vi "MarvinATP1.vi"() -> ()   [LabVIEW 2017]
uses:
  PCAN_Driver/ControlCAN.llb/InitFlag.ctl
  PCAN_Driver/ControlCAN.lvlib
  PCAN_Driver/ControlCAN.llb/Mode.ctl
  PCAN_Driver/ControlCAN.llb/Fliter.ctl
  PCAN_Driver/ControlCAN.llb/VCI_INIT_CONFIG.ctl
  PCAN_Driver/ControlCAN.llb/CAN Channel.ctl
  PCAN_Driver/ControlCAN.llb/DevType.ctl
panel:
  out "Auxiind":bool
  in  "Index":string="5"
  out "Array 2":dbl[](array[numeric])
  out "Array 3":string[](array[string])
  out "Array 4":dbl[](array[numeric])
  out "Array 5":dbl[](array[numeric])
  out "TempSensCalind":bool
  out "VisualInspectionResult":bool
  in  "Stop Burn-in":bool
  out "Burninind":bool
  out "TempControlind":bool
  out "TempAlg":bool=TRUE
  out "MotorTempind":bool
  out "SpeedStopind":bool
  out "VC15100-1 Vel":dbl
  out "VC15100-1 Cur":dbl
  out "VC1500-2 Vel":dbl
  out "VC15100-2":dbl
  out "EnableTestind":bool
  out "ComTestind":bool
  out "Ambient Temperature":dbl
  out "Motor Speed RPM":dbl
  out "Motor Stator Temp.":dbl
  out "Power transistor Heat sink Temp.":dbl
  in  "ATR":string[][](table)=[["Test Communication", "-", "-", "-", "-", ""], ["Set S/N", "-", "-", "-", "-", ""], ["Set Board Number", "-", "-", "-", "-", ""], [" ", "", "", "", "", ""], ["Test Communication", "-", "-", "-", "-", ""], ["Get S/N", "-", "-", "-", "", ""], ["Get Board Number", "-", "-", "-", "", ""], ["Get FW", "-", "-", "-", "", ""], ["Enable Motor", "", "", "", "", ""], ["Small position command", "", "", "", "", ""], ["Measure delta", "", "", "", "", ""], ["Velocity command", "", "", "", "", ""]]
  out "Pannel User Message":string
  out "Config_CANAT":T7 {"DevType" items=["USB-CAN"=3, "USB-CAN2"=4]; "CanIndex" items=["通道1", "通道2"]; "VCI_INIT_CONFIG"."Fliter" items=["接收所有类型"=3, "只接收标准帧"=4, "只接收扩展帧"=7]; "VCI_INIT_CONFIG"."Mode" items=["正常工作", "自测模式（环回）", "仅侦听模式"]; "VCI_INIT_CONFIG"."InitFlag" items=["使用Flash参数", "使用界面设置参数"]}
  in  "Stop Button":bool
  out "UUT":u8
  out "VISA resource name out":refnum<visa-resource-name>
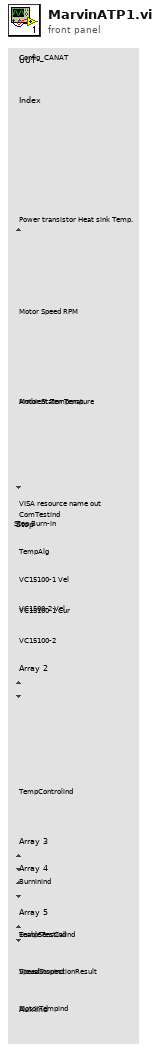
[diagram p1: front panel]
types:
  T1 = typedef "ControlCAN.lvlib/DevType.ctl" = u32
  T2 = typedef "ControlCAN.lvlib/CAN Channel.ctl" = u32
  T3 = typedef "ControlCAN.lvlib/VCI_INIT_CONFIG.ctl" = cluster{"AccCode":u32, "AccMask":u32, "InitFlag":T4, "Fliter":T5, "Timing0":u8, "Timing1":u8, "Mode":T6}
  T4 = typedef "ControlCAN.lvlib/InitFlag.ctl" = u32
  T5 = typedef "ControlCAN.lvlib/Fliter.ctl" = u8
  T6 = typedef "ControlCAN.lvlib/Mode.ctl" = u8
  T7 = cluster{"DevType":T1, "DevIndex":u32, "CanIndex":T2, "VCI_INIT_CONFIG":T3}
  T8 = enum16{"STOP", "VC15100-2", "RESET", "VC15100-1", "MD0"}
  T9 = enum8{"Enabled", "Disabled", "Disabled and Grayed Out"}
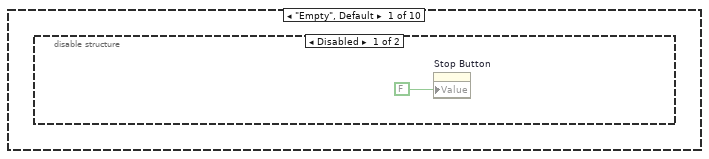
[diagram p2: hidden frame]
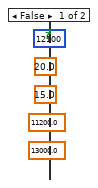
[diagram p6: hidden frame]
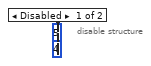
[diagram p7: hidden frame]
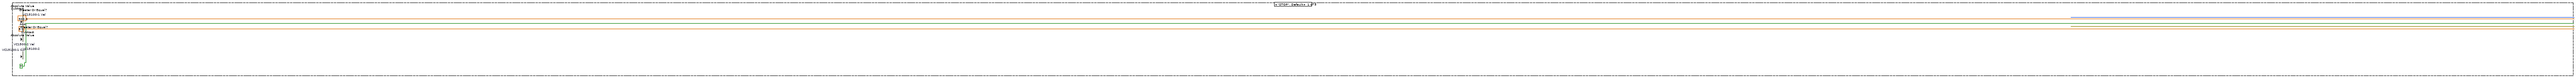
[diagram p8: hidden frame]
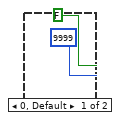
[diagram p9: hidden frame]
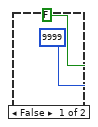
[diagram p10: hidden frame]
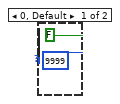
[diagram p11: hidden frame]
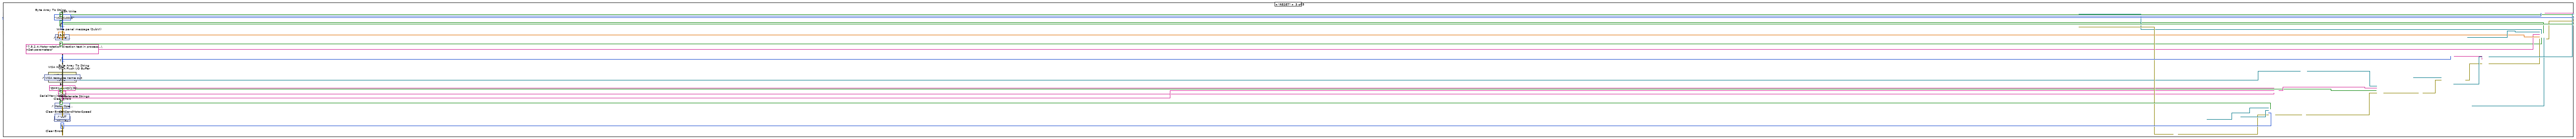
[diagram p13: hidden frame]
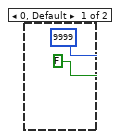
[diagram p15: hidden frame]
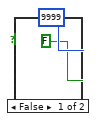
[diagram p16: hidden frame]
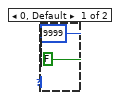
[diagram p17: hidden frame]
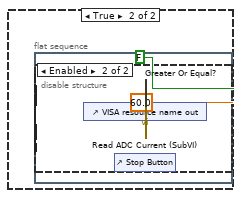
[diagram p18: hidden frame]
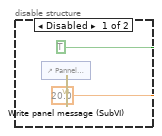
[diagram p19: hidden frame]
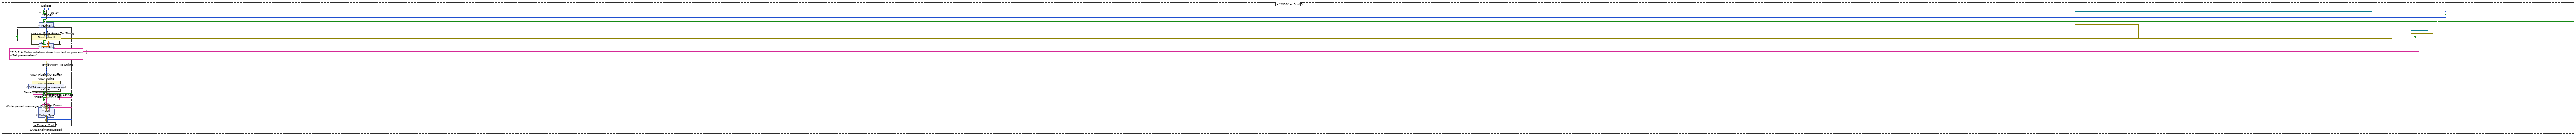
[diagram p20: hidden frame]
diagram:
  n1 = case shown="\"Auxiliary\"" {
    selector: _ -> [_ _ _ _ _ _ _ _ _ _]
    tunnel: _ -> [_ _ _ _ _ _ _ _ w1694 _]
    tunnel: _ -> [_ w34 w53 w705 w901 w1020 w1342 w1653 w1656 w1901]
    tunnel: _ -> [_ w14 w69 w710 w908 w1032 w1368 w1649 w1689 w1910]
    frame "Empty", Default {
      n2 = disable-structure shown="Disabled" {
        frame Disabled {
          n3 = property on="Stop Button" class="Bool (strict)"("Value"=FALSE ("Stop Button")) -> ()  [unwired: 2 in, 2 out]
        }
        frame Enabled {
        }
      }
    }
    frame "Com Test" {
      w11 = T9."Enabled" ("Disabled")
      w12 = T9."Disabled and Grayed Out" ("Disabled")
      w35 = 6 ("disabled index (col)")
      w4 = "7.4" ("Test Paragraph")
      n4 = control-ref of="Pannel User Message"() -> (w32:refnum<vi>)
      n5 = property on="Property Node" class="Bool (strict)"(error in=w14, "DisabledEnum"=w12) -> (error out=w13:errorcluster)  [unwired: 1 in, 1 out]
      n6 = property class="Str"(reference=w32, error in=w14, "Value"="7.4.Communication Test in process...") -> (error out=w3:errorcluster)  [unwired: 1 out]
      n7 = property on="Property Node" class="Bool (strict)"(error in=w13, "DisabledEnum"=w12) -> ()  [unwired: 1 in, 2 out]
      n8 = control-ref of="ATR"() -> (w5:refnum<vi>)
      n9 = call "Reset old test Values (SubVI).vi"("error in"=w3, "Atr in"=w5, "Test Paragraph"=w4) -> ("error out"=w2:errorcluster)  [unwired: 8 in]
      n10 = call "Table_ScrollaBarMarvin.vi"("error in"=w2, "Line to focus"=w4, "reference in"=w34) -> ("error out"=w33:errorcluster)  [unwired: 2 out]
      n11 = property on="Property Node" class="VISAName"() -> ("Value"=w29:refnum<visa-resource-name>)  [unwired: 2 in, 2 out]
      n12 = property on="Property Node" class="Str"() -> ("Value"=w18:string)  [unwired: 2 in, 2 out]
      n13 = control-ref of="UUT"() -> (w45:refnum<vi>)
      n14 = property class="Tbl (strict)"(reference=w34, error in=w33) -> (reference out=w22:refnum<vi>, error out=w49:errorcluster, "Value"=w6:string[][])
      n15 = Index Array(array=w6, index (col)=0 ("disabled index (col)")) -> (element=w50:string[])  [unwired: 1 in]
      n16 = call "Find_Number_LineMARVIN.vi"("Test Paragraph"=w4, "error in"=w49, "Row Headers[]"=w50) -> ("error out"=w47:errorcluster, "Line number"=w46:i32)  [unwired: 2 in, 2 out]
      n17 = call <vilib>:"Clear Errors.vi"("error in (no error)"=w47) -> ("error out"=w8:errorcluster)  [unwired: 5 in, 1 out]
      n18 = call "Time Delay"("error in (no error)"=w8) -> ("error out"=w7:errorcluster)  [unwired: 10 in]
      n19 = VISA Flush I/O Buffer(VISA resource name=w29, error in (no error)=w7) -> (VISA resource name out=w27:refnum<visa-resource-name>, error out=w28:errorcluster)  [unwired: 1 in]
      n20 = call "SerialMarvinMod.vi"("error in (no error)"=w28, "write buffer"="VR\r\n", "VISA resource name"=w27) -> ("error out"=w21:errorcluster, "read buffer"=w24:string)  [unwired: 7 in]
      n21 = Equal?(x=w18, y=w24) -> (x = y?=w16:bool)
      n22 = Increment(x=w46) -> (x+1=w26:i32)
      n23 = Increment(x=w26) -> (x+1=w37:i32)
      n24 = Replace Array Subset(array=w6, new element=w24, index (row)=w26, index (col)=5 ("disabled index (col)")) -> (w23:string[][])
      n25 = property class="Tbl (strict)"(reference=w22, error in=w21, "Value"=w23) -> (error out=w20:errorcluster)  [unwired: 1 out]
      n26 = call "PassOrFail (SubVI).vi"("disabled index (col)"=w35, "index (row)"=w26, "error in (no error)"=w20, "Boolean"=w16, "Table in"=w34) -> ("error out"=w19:errorcluster)  [unwired: 6 in]
      n27 = property class="DigNum (strict)"(reference=w45, error in=w19) -> (error out=w36:errorcluster, "Value"=w44:u8)  [unwired: 1 out]
      n28 = Equal?(x=w44, y=u8 47) -> (x = y?=w40:bool)
      n29 = Equal?(x=w44, y=u8 63) -> (x = y?=w39:bool)
      n30 = Equal?(x=w44, y=u8 95) -> (x = y?=w38:bool)
      n31 = Compound Arithmetic op=OR(w40, w39, w38) -> (w17:bool)
      n32 = call "PassOrFail (SubVI).vi"("disabled index (col)"=w35, "index (row)"=w37, "error in (no error)"=w36, "Boolean"=w17, "Table in"=w34) -> ("error out"=w9:errorcluster)  [unwired: 6 in]
      n33 = property on="Property Node" class="Bool (strict)"(error in=w9, "DisabledEnum"=w11) -> (error out=w10:errorcluster)  [unwired: 1 in, 1 out]
      n34 = property on="Property Node" class="Bool (strict)"(error in=w10, "DisabledEnum"=w11) -> ()  [unwired: 1 in, 2 out]
      n35 = And(x=w17, y=w16) -> (x .and. y?=→"ComTestind":bool)
    }
    frame "Enable Test" {
      w68 = T9."Enabled" ("Disabled")
      w71 = T9."Disabled and Grayed Out" ("Disabled")
      w52 = "7.5.2" ("Test Paragraph")
      n36 = control-ref of="Pannel User Message"() -> (w87:refnum<vi>)
      n37 = property on="Property Node" class="Bool (strict)"(error in=w69, "DisabledEnum"=w71) -> (error out=w70:errorcluster)  [unwired: 1 in, 1 out]
      n38 = property class="Str"(reference=w87, error in=w69, "Value"="7.5.2.Enable Test") -> (error out=w86:errorcluster)  [unwired: 1 out]
      n39 = property on="Property Node" class="Bool (strict)"(error in=w70, "DisabledEnum"=w71) -> ()  [unwired: 1 in, 2 out]
      n40 = call "Table_ScrollaBarMarvin.vi"("error in"=w86, "Line to focus"=w52, "reference in"=w53) -> ("error out"=w125:errorcluster)  [unwired: 2 out]
      n41 = call "Reset old test Values (SubVI).vi"("error in"=w125, "Atr in"=w53, "Test Paragraph"=w52) -> ("error out"=w54:errorcluster)  [unwired: 8 in]
      n42 = property class="Tbl (strict)"(reference=w53, error in=w54) -> (error out=w127:errorcluster, "Value"=w128:string[][])  [unwired: 1 out]
      n43 = control-ref of="VISA resource name out"() -> (w98:refnum<vi>)
      n44 = property on="Property Node" class="Str"() -> ("Value"=w62:string)  [unwired: 2 in, 2 out]
      n45 = control-ref of="Stop Button"() -> (w64:refnum<vi>)
      n46 = control-ref of="Config_CANAT"() -> (w80:refnum<vi>)
      n47 = control-ref of="UUT"() -> (w81:refnum<vi>)
      n48 = Initialize Array(FALSE, 14 ("dimension size")) -> (w110:bool[])
      n49 = Build Array (concatenate)(w110, bool[] [FALSE, FALSE, FALSE, FALSE, FALSE, FALSE, FALSE] ("array")) -> (w111:bool[])
      n50 = Boolean Array To Number(Boolean array=w111) -> (number=w109:u32)
      n51 = To Unsigned Long Integer(number=w109) -> (unsigned 32bit integer=w100:u32)
      n52 = Split Number(x=w100) -> (hi(x)=w105:u16, lo(x)=w106:u16)
      n53 = Split Number(x=w106) -> (hi(x)=w104:u8, lo(x)=w103:u8)
      n54 = Index Array(array=w128, index (col)=0 ("disabled index (col)")) -> (element=w129:string[])  [unwired: 1 in]
      n55 = Equal?(x=w62, y="EBAY") -> (x = y?=w60:bool)
      n56 = case shown="True" w60 {
        tunnel: [u16 12100 ("Motor Speed RPM") u16 15100 ("Motor Speed RPM")] -> w59
        tunnel: [11200.0 ("y") 14800.0 ("y")] -> w58
        tunnel: [13000.0 ("y") 16000.0 ("y")] -> w57
        tunnel: [20.0 ("y") 48.0 ("y")] -> w56
        tunnel: [15.0 ("y") 40.0 ("y")] -> w55
        frame False {
        }
        frame True {
        }
      }
      n57 = call "Find_Number_LineMARVIN.vi"("Test Paragraph"=w52, "error in"=w127, "Row Headers[]"=w129) -> ("error out"=w63:errorcluster, "Line number"=w124:i32)  [unwired: 2 in, 2 out]
      n58 = for {
        tunnel: w53 -> [w663]
        tunnel: w124 -> [w653]
        tunnel: u16[] [5000, 0, 5000] -> [w628] mode=indexing
        tunnel: [w651] -> w122
        tunnel: w63 -> [w629]
        tunnel: bool[] [TRUE, FALSE, TRUE] -> [w627] mode=indexing
        tunnel: bool[] [TRUE, TRUE, TRUE] -> [w626] mode=indexing
        tunnel: [w625] -> w77 mode=indexing
        i -> [w655]
        w656 = 200.0 ("y")
        n59 = control-ref of="VISA resource name out"() -> (w648:refnum<vi>)
        n60 = control-ref of="Config_CANAT"() -> (w670:refnum<vi>)
        n61 = while {
          tunnel: [w675] -> w665
          tunnel: [w692] -> w664
          tunnel: w622 -> [w691]
          tunnel: w624 -> [w689]
          stop <- w674 stop-if-true
          w686 = 15.0 ("y")
          n62 = control-ref of="Motor Speed RPM"() -> (w693:refnum<vi>)
          n63 = control-ref of="Pannel User Message"() -> (w687:refnum<vi>)
          n64 = flat-sequence {
            tunnel: [w694] -> w690
            frame #0 {
              n65 = call <vilib>:"High Resolution Relative Seconds.vi"() -> ("relative seconds"=w694:dbl)
            }
          }
          n66 = property on="Stop Button" class="Bool (strict)"() -> ("Value"=w673:bool)  [unwired: 2 in, 2 out]
          n67 = Subtract(x=w690, y=w689) -> (x-y=w685:dbl)
          n68 = Greater Or Equal?(x=w685, y=w686) -> (x >= y?=w688:bool)
          n69 = Compound Arithmetic op=OR(w673, w688) -> (w674:bool)
          n70 = Subtract(x=w686, y=w685) -> (x-y=w677:dbl)
          n71 = Number To Fractional String(number=w677, precision (6)=i16 2) -> (F-format string=w683:string)  [unwired: 2 in]
          n72 = property class="DigNum (strict)"(reference=w693, error in=w691) -> (error out=w692:errorcluster, "Value"=w675:dbl)  [unwired: 1 out]
          n73 = Number To Decimal String(number=w675) -> (decimal integer string=w684:string)  [unwired: 1 in]
          n74 = Concatenate Strings("7.5.2.Enable Test in process...\nRemained Time: " ("string"), w683, "  sec." ("string"), "\r\n", "Motor speed [rpm]: " ("string"), w684) -> (w678:string)
          n75 = property class="Str"(reference=w687, "Value"=w678) -> ()  [unwired: 1 in, 2 out]
        }
        n76 = Add(x=w628, y=w656) -> (x+y=w658:dbl)
        n77 = Increment(x=w655) -> (x+1=w654:i32)
        n78 = flat-sequence {
          tunnel: [w672] -> w624
          tunnel: w623 -> [w671]
          tunnel: [w671] -> w622
          frame #0 {
            n79 = call <vilib>:"High Resolution Relative Seconds.vi"() -> ("relative seconds"=w672:dbl)
          }
        }
        n80 = Subtract(x=w628, y=w656) -> (x-y=w657:dbl)
        n81 = In Range and Coerce(upper limit=w658, x=w665, lower limit=w657) -> (In Range?=w625:bool)  [unwired: 1 out]
        n82 = Add(x=w653, y=w654) -> (x+y=w650:i32)
        n83 = case shown="True" w627 {
          tunnel: [bool[] [FALSE, FALSE, FALSE, FALSE, FALSE, FALSE, FALSE] ("array") bool[] [FALSE, FALSE, FALSE, TRUE, FALSE, FALSE, FALSE] ("array")] -> w635
          frame False {
          }
          frame True {
          }
        }
        n84 = call <vilib>:"Clear Errors.vi"("error in (no error)"=w664) -> ("error out"=w621:errorcluster)  [unwired: 5 in, 1 out]
        n85 = call "PassOrFail (SubVI).vi"("disabled index (col)"=6, "index (row)"=w650, "error in (no error)"=w621, "Boolean"=w625, "Table in"=w663) -> ("error out"=w667:errorcluster)  [unwired: 6 in]
        n86 = property class="Tbl (strict)"(reference=w663, error in=w667) -> (reference out=w659:refnum<vi>, error out=w668:errorcluster, "Value"=w660:string[][])
        n87 = Build Array (concatenate)(bool[] [FALSE, FALSE, FALSE, TRUE, FALSE, FALSE, FALSE, FALSE, FALSE, FALSE, FALSE, FALSE, FALSE, FALSE] ("array"), w635) -> (w636:bool[])
        n88 = Boolean Array To Number(Boolean array=w636) -> (number=w637:u32)
        n89 = To Unsigned Long Integer(number=w637) -> (unsigned 32bit integer=w646:u32)
        n90 = Split Number(x=w646) -> (hi(x)=w641:u16, lo(x)=w640:u16)
        n91 = Split Number(x=w640) -> (hi(x)=w642:u8, lo(x)=w643:u8)
        n92 = Number To Fractional String(number=w665, precision (6)=i16 2) -> (F-format string=w662:string)  [unwired: 2 in]
        n93 = Replace Array Subset(array=w660, new element=w662, index (row)=w650, index (col)=5 ("disabled index (col)")) -> (w661:string[][])
        n94 = property class="Tbl (strict)"(reference=w659, error in=w668, "Value"=w661) -> (error out=w651:errorcluster)  [unwired: 1 out]
        n95 = property class="VISAName"(reference=w648, error in=w629) -> (error out=w649:errorcluster, "Value"=w639:refnum<visa-resource-name>)  [unwired: 1 out]
        n96 = Split Number(x=w641) -> (hi(x)=w644:u8, lo(x)=w645:u8)
        n97 = Build Array(u8 75, u8 0 ("element"), u8 4 ("Length"), u8 2, w643, w642, w645, w644) -> (w638:u8[])
        n98 = Byte Array To String(unsigned byte array=w638) -> (string=w647:string)
        n99 = VISA Write(VISA resource name=w639, write buffer=w647, error in (no error)=w649) -> (error out=w630:errorcluster)  [unwired: 2 out]
        n100 = case shown="True" w626 {
          tunnel: w670 -> [_ w700]
          tunnel: [w695 w699] -> w623
          tunnel: w630 -> [w695 w697]
          frame False {
          }
          frame True {
            n101 = control-ref of="UUT"() -> (w701:refnum<vi>)
            n102 = call "CANSendMotorSpeed.vi"("Remote"=TRUE, "error in (no error)"=w697, "Motor Speed RPM"=u16 5000, "UUT"=w701, "Cluster in"=w700) -> ("error out"=w699:errorcluster)  [unwired: 6 in]
          }
        }
      }
      n103 = And Array Elements(Boolean array=w77) -> (logical AND=w76:bool)
      n104 = Split Number(x=w105) -> (hi(x)=w102:u8, lo(x)=w101:u8)
      n105 = Build Array(u8 75, u8 0 ("element"), u8 4 ("Length"), u8 2, w103, w104, w101, w102) -> (w108:u8[])
      n106 = Byte Array To String(unsigned byte array=w108) -> (string=w99:string)
      n107 = call <vilib>:"Clear Errors.vi"("error in (no error)"=w122) -> ("error out"=w73:errorcluster)  [unwired: 5 in, 1 out]
      n108 = disable-structure shown="Enabled" {
        disable-tunnel: w73 -> [w162 w618]
        disable-tunnel: [w161 w617] -> w79
        disable-tunnel: [w160 w619] -> w75
        disable-tunnel: T8."MD0" -> [w159 _]
        disable-tunnel: w64 -> [w158 _]
        disable-tunnel: w59 -> [w157 _]
        disable-tunnel: w58 -> [w156 _]
        disable-tunnel: w57 -> [w155 _]
        disable-tunnel: w56 -> [w154 _]
        disable-tunnel: w55 -> [w153 _]
        frame Enabled {
          n109 = while {
            tunnel: [w174] -> w160
            tunnel: w162 -> [w176]
            tunnel: [w175] -> w161
            shift-right: [w172] -> _
            shift-left: w159 -> [w173]
            tunnel: w158 -> [w168]
            tunnel: w157 -> [w167]
            tunnel: w156 -> [w166]
            tunnel: w155 -> [w165]
            tunnel: w154 -> [w164]
            tunnel: w153 -> [w163]
            stop <- w170 stop-if-true
            n110 = case shown="\"VC15100-2\"" w173 {
              selector: w173 -> [w190 _ _ _ _]
              tunnel: w176 -> [w191 w219 w373 w413 w579]
              tunnel: [w191 w212 w379 w407 w578] -> w175
              tunnel: [w183 FALSE FALSE FALSE FALSE] -> w174
              tunnel: [w190 T8."STOP" T8."VC15100-2" w399 w582] -> w172
              tunnel: [TRUE FALSE FALSE FALSE FALSE] -> w171
              tunnel: w168 -> [_ w198 w357 w393 w573]
              tunnel: w167 -> [_ w197 _ _ _]
              tunnel: w166 -> [_ w196 _ _ _]
              tunnel: w165 -> [_ w195 _ _ _]
              tunnel: w164 -> [_ w194 _ w391 _]
              tunnel: w163 -> [_ w193 _ w392 _]
              frame "STOP", Default {
                n111 = property on="VC15100-1 Vel" class="DigNum (strict)"() -> ("Value"=w182:dbl)  [unwired: 2 in, 2 out]
                n112 = property on="VC1500-2 Vel" class="DigNum (strict)"() -> ("Value"=w181:dbl)  [unwired: 2 in, 2 out]
                n113 = Subtract(x=w182, y=w181) -> (x-y=w180:dbl)
                n114 = Absolute Value(x=w180) -> (abs(x)=w179:dbl)
                n115 = Greater Or Equal?(x=w179, y=500.0) -> (x >= y?=w177:bool)
                n116 = property on="VC15100-2" class="DigNum (strict)"() -> ("Value"=w189:dbl)  [unwired: 2 in, 2 out]
                n117 = property on="VC15100-1 Cur" class="DigNum (strict)"() -> ("Value"=w188:dbl)  [unwired: 2 in, 2 out]
                n118 = Subtract(x=w189, y=w188) -> (x-y=w185:dbl)
                n119 = Absolute Value(x=w185) -> (abs(x)=w184:dbl)
                n120 = Greater Or Equal?(x=w184, y=5.0) -> (x >= y?=w186:bool)
                n121 = And(x=w177, y=w186) -> (x .and. y?=w183:bool)
              }
              frame "VC15100-2" {
                n122 = control-ref of="VISA resource name out"() -> (w214:refnum<vi>)
                n123 = property on="Property Node" class="DigNum (strict)"() -> ("Value"=w207:dbl)  [unwired: 2 in, 2 out]
                n124 = flat-sequence {
                  tunnel: [w313] -> w218
                  tunnel: w217 -> [w312]
                  tunnel: [w312] -> w216
                  frame #0 {
                    n125 = call <vilib>:"High Resolution Relative Seconds.vi"() -> ("relative seconds"=w313:dbl)
                  }
                }
                n126 = control-ref of="Config_CANAT"() -> (w221:refnum<vi>)
                n127 = control-ref of="UUT"() -> (w220:refnum<vi>)
                n128 = call <vilib>:"Clear Errors.vi"("error in (no error)"=w216) -> ("error out"=w206:errorcluster)  [unwired: 5 in, 1 out]
                n129 = while {
                  tunnel: w218 -> [w337]
                  tunnel: w206 -> [w331]
                  tunnel: [w332] -> w213
                  tunnel: [w330] -> w211
                  tunnel: w198 -> [w318]
                  tunnel: w196 -> [w315]
                  tunnel: w195 -> [w314]
                  stop <- w335 stop-if-true
                  w316 = "7.5.2.4.Motor rotation direction test in process..." ("string")
                  n130 = control-ref of="Motor Speed RPM"() -> (w317:refnum<vi>)
                  n131 = control-ref of="Pannel User Message"() -> (w326:refnum<vi>)
                  n132 = property class="DigNum (strict)"(reference=w317, error in=w331) -> (error out=w332:errorcluster, "Value"=w321:dbl)  [unwired: 1 out]
                  "VC1500-2 Vel" <- w321
                  n133 = Number To Fractional String(number=w321, precision (6)=i16 2) -> (F-format string=w325:string)  [unwired: 2 in]
                  n134 = Concatenate Strings(w316, "\r\n", "Motor speed [rpm]: " ("string"), w325) -> (w320:string)
                  n135 = property class="Str"(reference=w326, "Value"=w320) -> ()  [unwired: 1 in, 2 out]
                  n136 = Greater Or Equal?(x=w321, y=w315) -> (x >= y?=w329:bool)
                  n137 = call <vilib>:"High Resolution Relative Seconds.vi"() -> ("relative seconds"=w338:dbl)
                  n138 = Subtract(x=w338, y=w337) -> (x-y=w333:dbl)
                  n139 = Less Or Equal?(x=w321, y=w314) -> (x <= y?=w328:bool)
                  n140 = And(x=w329, y=w328) -> (x .and. y?=w327:bool)
                  n141 = case shown="True" w327 {
                    selector: w327 -> [w339 w344]
                    tunnel: [w339 w343] -> w330
                    tunnel: w316 -> [_ w342]
                    tunnel: w318 -> [_ w341]
                    tunnel: w317 -> [_ w340]
                    frame False {
                    }
                    frame True {
                      n142 = flat-sequence {
                        tunnel: w344 -> [w351]
                        tunnel: [w351] -> w343
                        tunnel: w342 -> [w348]
                        tunnel: w341 -> [w347]
                        tunnel: w340 -> [w346]
                        frame #0 {
                          n143 = control-ref of="Pannel User Message"() -> (w349:refnum<vi>)
                          n144 = call "Write panel message (SubVI).vi"(4:"rpm"=w346, 5:"rpm"=TRUE ("rpm"), "Stop"=w347, "Time to wait"=20.0, "Strin"=w348, "String in"=w349) -> ()  [unwired: 5 in, 1 out]
                        }
                      }
                    }
                  }
                  n145 = Greater Or Equal?(x=w333, y=60.0) -> (x >= y?=w334:bool)
                  n146 = property on="Stop Button" class="Bool (strict)"() -> ("Value"=w319:bool)  [unwired: 2 in, 2 out]
                  n147 = Compound Arithmetic op=OR(w330, w334, w319) -> (w335:bool)
                }
                n148 = for {
                  N: 10 -> [_]
                  tunnel: w214 -> [w234]
                  tunnel: [w223] -> w209 mode=indexing
                  shift-right: [w224] -> w212
                  shift-left: w213 -> [w233]
                  tunnel: w193 -> [w222]
                  n149 = flat-sequence {
                    tunnel: w232 -> [w236]
                    tunnel: [w236] -> w229
                    tunnel: [w235] -> w228
                    frame #0 {
                      n150 = call <vilib>:"High Resolution Relative Seconds.vi"() -> ("relative seconds"=w235:dbl)
                    }
                  }
                  n151 = Byte Array To String(unsigned byte array=u8[] [75, 0, 4, 17, 0, 0, 0, 0] ("appended array")) -> (string=w231:string)
                  n152 = property class="VISAName"(reference=w234, error in=w233) -> (error out=w225:errorcluster, "Value"=w226:refnum<visa-resource-name>)  [unwired: 1 out]
                  n153 = VISA Write(VISA resource name=w226, write buffer=w231, error in (no error)=w225) -> (VISA resource name out=w230:refnum<visa-resource-name>, error out=w232:errorcluster)  [unwired: 1 out]
                  n154 = while {
                    tunnel: w230 -> [w250]
                    tunnel: w229 -> [w249]
                    tunnel: [w248] -> _
                    tunnel: [w247] -> w224
                    tunnel: w228 -> [w245]
                    tunnel: [w239] -> w223
                    tunnel: w222 -> [w237]
                    stop <- w241 stop-if-true
                    n155 = VISA Read(VISA resource name=w250, byte count=u32 1, error in (no error)=w249) -> (VISA resource name out=w252:refnum<visa-resource-name>, read buffer=w253:string, error out=w251:errorcluster)  [unwired: 1 out]
                    n156 = String To Byte Array(string=w253) -> (unsigned byte array=w256:u8[])
                    n157 = Index Array(array=w256, index=0) -> (element=w254:u8)
                    n158 = case shown="75" w254 {
                      tunnel: [w261 w266] -> w247
                      tunnel: w252 -> [w260 w275]
                      tunnel: w251 -> [w261 w274]
                      tunnel: [w260 w267] -> w248
                      tunnel: [u32 9999 w264] -> w239
                      tunnel: [FALSE w263] -> w240
                      tunnel: w237 -> [_ w262]
                      frame 0, Default {
                      }
                      frame 75 {
                        n159 = VISA Read(VISA resource name=w275, byte count=u32 3, error in (no error)=w274) -> (VISA resource name out=w270:refnum<visa-resource-name>, read buffer=w278:string, error out=w269:errorcluster)  [unwired: 1 out]
                        n160 = String To Byte Array(string=w278) -> (unsigned byte array=w268:u8[])
                        n161 = Index Array(array=w268, index #1=0 ("index")) -> (element #1=w273:u8, element #2=w271:u8)  [unwired: 2 in, 1 out]
                        n162 = Equal?(x=u8 0, y=w273) -> (x = y?=w272:bool)
                        n163 = case shown="True" w272 {
                          tunnel: [w281 w289] -> w266
                          tunnel: w271 -> [_ w296]
                          tunnel: w270 -> [w282 w295]
                          tunnel: w269 -> [w281 w294]
                          tunnel: w268 -> [_ w293]
                          tunnel: [w282 w291] -> w267
                          tunnel: [u32 9999 w285] -> w264
                          tunnel: [FALSE w284] -> w263
                          tunnel: w262 -> [_ w283]
                          frame False {
                          }
                          frame True {
                            n164 = VISA Read(VISA resource name=w295, byte count=w296, error in (no error)=w294) -> (VISA resource name out=w291:refnum<visa-resource-name>, read buffer=w290:string, error out=w289:errorcluster)  [unwired: 1 out]
                            n165 = String To Byte Array(string=w290) -> (unsigned byte array=w292:u8[])
                            n166 = Insert Into Array(array=w293, new element=w292) -> (w286:u8[])  [unwired: 1 in]
                            n167 = Index Array(array=w286, index #1=0 ("index")) -> (element #3=w287:u8)  [unwired: 2 in, 2 out]
                            n168 = case shown="15..19" w287 {
                              tunnel: w286 -> [_ w310]
                              tunnel: [u32 9999 w300] -> w285
                              tunnel: [FALSE w301] -> w284
                              tunnel: w283 -> [_ w299]
                              frame 0, Default {
                              }
                              frame 15..19 {
                                n169 = Index Array(array=w310, index #1=3 ("index")) -> (element #1=w309:u8, element #2=w308:u8, element #3=w307:u8, element #4=w306:u8)  [unwired: 3 in]
                                n170 = Join Numbers(hi=w306, lo=w307) -> ((hi.lo)=w304:u16)
                                n171 = Join Numbers(hi=w308, lo=w309) -> ((hi.lo)=w305:u16)
                                n172 = Join Numbers(hi=w304, lo=w305) -> ((hi.lo)=w302:u32)
                                n173 = Multiply(x=0.02003173828125, y=w302) -> (x*y=w300:dbl)
                                n174 = Greater Or Equal?(x=w300, y=w299) -> (x >= y?=w301:bool)
                              }
                            }
                          }
                        }
                      }
                    }
                    n175 = call <vilib>:"High Resolution Relative Seconds.vi"() -> ("relative seconds"=w246:dbl)
                    n176 = Subtract(x=w246, y=w245) -> (x-y=w244:dbl)
                    n177 = Greater Or Equal?(x=w244, y=2.0) -> (x >= y?=w242:bool)
                    n178 = property on="Stop Button" class="Bool (strict)"() -> ("Value"=w238:bool)  [unwired: 2 in, 2 out]
                    n179 = Compound Arithmetic op=OR(w238, w242, w240) -> (w241:bool)
                  }
                }
                n180 = Add Array Elements(numeric array=w209) -> (sum=w201:dbl)
                n181 = Divide(x=w201, y=10.0 ("x")) -> (x/y=w200:dbl)
                n182 = Subtract(x=w200, y=w207) -> (x-y=w208:dbl)
                "VC15100-2" <- w208
                n183 = call "CANSendMotorSpeed.vi"("Remote"=TRUE, "error in (no error)"=w219, "Motor Speed RPM"=w197, "UUT"=w220, "Cluster in"=w221) -> ("error out"=w217:errorcluster)  [unwired: 6 in]
                n184 = Greater Or Equal?(x=w208, y=w194) -> (x >= y?=w210:bool)
                n185 = And(x=w210, y=w211) -> ()  [unwired: 1 out]
              }
              frame "RESET" {
                # "Venable + Power ON"
                # "Venable + Power OFF"
                n186 = control-ref of="VISA resource name out"() -> (w387:refnum<vi>)
                n187 = property on="Property Node" class="VISAName"() -> ("Value"=w371:refnum<visa-resource-name>)  [unwired: 2 in, 2 out]
                n188 = control-ref of="Config_CANAT"() -> (w374:refnum<vi>)
                n189 = control-ref of="Motor Speed RPM"() -> (w355:refnum<vi>)
                n190 = control-ref of="UUT"() -> (w375:refnum<vi>)
                n191 = control-ref of="Pannel User Message"() -> (w362:refnum<vi>)
                n192 = Byte Array To String(unsigned byte array=u8[] [75, 0, 4, 2, 0, 0, 2, 0]) -> (string=w385:string)
                n193 = Byte Array To String(unsigned byte array=u8[] [75, 0, 4, 2, 0, 0, 18, 0]) -> (string=w388:string)
                n194 = VISA Flush I/O Buffer(VISA resource name=w371) -> (VISA resource name out=w372:refnum<visa-resource-name>)  [unwired: 2 in, 1 out]
                n195 = Concatenate Strings("EP=1\r\nMD[1]=" ("write buffer"), "1" ("string"), "\r\n" ("string")) -> (w370:string)
                n196 = call <vilib>:"Clear Errors.vi"("error in (no error)"=w373) -> ("error out"=w353:errorcluster)  [unwired: 5 in, 1 out]
                n197 = call "CANSendMotorSpeed.vi"("Remote"=TRUE, "error in (no error)"=w353, "Motor Speed RPM"=u16 0, "UUT"=w375, "Cluster in"=w374) -> ("error out"=w365:errorcluster)  [unwired: 6 in]
                n198 = call <vilib>:"Clear Errors.vi"("error in (no error)"=w365) -> ("error out"=w352:errorcluster)  [unwired: 5 in, 1 out]
                n199 = call "SerialMarvinMod.vi"("error in (no error)"=w352, "Clear Log"=FALSE, "write buffer"=w370, "VISA resource name"=w372) -> ("error out"=w364:errorcluster)  [unwired: 6 in, 1 out]
                n200 = call <vilib>:"Clear Errors.vi"("error in (no error)"=w364) -> ("error out"=w363:errorcluster)  [unwired: 5 in, 1 out]
                n201 = property class="VISAName"(reference=w387, error in=w363) -> (error out=w386:errorcluster, "Value"=w389:refnum<visa-resource-name>)  [unwired: 1 out]
                n202 = VISA Write(VISA resource name=w389, write buffer=w388, error in (no error)=w386) -> (VISA resource name out=w384:refnum<visa-resource-name>, error out=w360:errorcluster)  [unwired: 1 out]
                n203 = call "Write panel message (SubVI).vi"(4:"rpm"=w355, 5:"rpm"=FALSE ("rpm"), "PrintTime"=TRUE, "Stop"=w357, "error in (no error)"=w360, "Time to wait"=15.0, "Strin"="7.5.2.4.Motor rotation direction test in process...\nSet parameters" ("string"), "String in"=w362) -> ("error out"=w359:errorcluster)  [unwired: 3 in]
                n204 = VISA Write(VISA resource name=w384, write buffer=w385, error in (no error)=w359) -> (error out=w379:errorcluster)  [unwired: 2 out]
              }
              frame "VC15100-1" {
                n205 = property on="Property Node" class="DigNum (strict)"() -> ("Value"=w403:dbl)  [unwired: 2 in, 2 out]
                n206 = control-ref of="Config_CANAT"() -> (w415:refnum<vi>)
                n207 = control-ref of="UUT"() -> (w414:refnum<vi>)
                n208 = flat-sequence {
                  tunnel: [w508] -> w411
                  tunnel: w410 -> [w507]
                  tunnel: [w507] -> w409
                  frame #0 {
                    n209 = call <vilib>:"High Resolution Relative Seconds.vi"() -> ("relative seconds"=w508:dbl)
                  }
                }
                n210 = call "CANSendMotorSpeed.vi"("Remote"=TRUE, "error in (no error)"=w413, "Motor Speed RPM"=u16 15100, "UUT"=w414, "Cluster in"=w415) -> ("error out"=w410:errorcluster)  [unwired: 6 in]
                n211 = call <vilib>:"Clear Errors.vi"("error in (no error)"=w409) -> ("error out"=w402:errorcluster)  [unwired: 5 in, 1 out]
                n212 = while {
                  tunnel: w411 -> [w533]
                  tunnel: w402 -> [w528]
                  tunnel: [w527] -> w406
                  tunnel: w393 -> [w515]
                  tunnel: [w509] -> w390
                  stop <- w531 stop-if-true
                  w512 = "7.5.2.4.Motor rotation direction test in process..." ("string")
                  n213 = control-ref of="Motor Speed RPM"() -> (w513:refnum<vi>)
                  n214 = control-ref of="Pannel User Message"() -> (w519:refnum<vi>)
                  n215 = call <vilib>:"High Resolution Relative Seconds.vi"() -> ("relative seconds"=w534:dbl)
                  n216 = Subtract(x=w534, y=w533) -> (x-y=w529:dbl)
                  n217 = Greater Or Equal?(x=w529, y=60.0) -> (x >= y?=w530:bool)
                  n218 = property on="Stop Button" class="Bool (strict)"() -> ("Value"=w514:bool)  [unwired: 2 in, 2 out]
                  n219 = property class="DigNum (strict)"(reference=w513, error in=w528) -> (error out=w510:errorcluster, "Value"=w517:dbl)  [unwired: 1 out]
                  "VC15100-1 Vel" <- w517
                  n220 = Number To Fractional String(number=w517, precision (6)=i16 2) -> (F-format string=w518:string)  [unwired: 2 in]
                  n221 = Concatenate Strings(w512, "\r\n", "Motor speed [rpm]: " ("string"), w518) -> (w516:string)
                  n222 = property class="Str"(reference=w519, "Value"=w516) -> ()  [unwired: 1 in, 2 out]
                  n223 = Greater Or Equal?(x=w517, y=12800.0) -> (x >= y?=w526:bool)
                  n224 = Less Or Equal?(x=w517, y=16000.0) -> (x <= y?=w525:bool)
                  n225 = And(x=w526, y=w525) -> (x .and. y?=w523:bool)
                  n226 = case shown="False" w523 {
                    selector: w523 -> [w543 w551]
                    tunnel: [w543 w550] -> w527
                    tunnel: w512 -> [_ w549]
                    tunnel: w515 -> [_ w548]
                    tunnel: w513 -> [_ w547]
                    tunnel: [w539 w546] -> w511
                    tunnel: w510 -> [w536 w545]
                    tunnel: [w537 w544] -> w509
                    frame False {
                      n227 = control-ref of="VISA resource name out"() -> (w542:refnum<vi>)
                      n228 = control-ref of="Stop Button"() -> (w541:refnum<vi>)
                      n229 = call "Read ADC Current (SubVI).vi"("error out"=w536, "Bool Refnum"=w541, "VISAResourceName in"=w542) -> ("error out 2"=w537:errorcluster, "Result"=w540:dbl)  [unwired: 7 in]
                      n230 = Greater Or Equal?(x=w540, y=60.0) -> (x >= y?=w539:bool)
                    }
                    frame True {
                      n231 = flat-sequence {
                        tunnel: w551 -> [_]
                        tunnel: [FALSE] -> w550
                        tunnel: w549 -> [w558]
                        tunnel: w548 -> [w557]
                        tunnel: w547 -> [w556]
                        tunnel: [w555] -> w546
                        tunnel: w545 -> [w553]
                        tunnel: [w552] -> w544
                        frame #0 {
                          n232 = disable-structure shown="Enabled" {
                            disable-tunnel: w558 -> [w562 _]
                            disable-tunnel: w557 -> [w561 _]
                            disable-tunnel: w556 -> [w559 _]
                            disable-tunnel: [_ w567] -> w555
                            disable-tunnel: w553 -> [_ w566]
                            disable-tunnel: [_ w565] -> w552
                            frame Disabled {
                              n233 = control-ref of="Pannel User Message"() -> (w564:refnum<vi>)
                              n234 = call "Write panel message (SubVI).vi"(4:"rpm"=w559, 5:"rpm"=TRUE ("rpm"), "Stop"=w561, "Time to wait"=20.0, "Strin"=w562, "String in"=w564) -> ()  [unwired: 5 in, 1 out]
                            }
                            frame Enabled {
                              n235 = control-ref of="VISA resource name out"() -> (w571:refnum<vi>)
                              n236 = control-ref of="Stop Button"() -> (w570:refnum<vi>)
                              n237 = call "Read ADC Current (SubVI).vi"("error out"=w566, "Bool Refnum"=w570, "VISAResourceName in"=w571) -> ("error out 2"=w565:errorcluster, "Result"=w568:dbl)  [unwired: 7 in]
                              n238 = Greater Or Equal?(x=w568, y=60.0) -> (x >= y?=w567:bool)
                            }
                          }
                        }
                      }
                    }
                  }
                  n239 = Compound Arithmetic op=OR(w527, w530, w514, w511) -> (w531:bool)
                }
                n240 = for {
                  N: 10 -> [_]
                  tunnel: [w419] -> w397 mode=indexing
                  tunnel: [T8."RESET"] -> w399
                  tunnel: w390 -> [w429]
                  tunnel: [w420] -> w407
                  tunnel: w392 -> [w417]
                  n241 = control-ref of="VISA resource name out"() -> (w416:refnum<vi>)
                  n242 = flat-sequence {
                    tunnel: w428 -> [w431]
                    tunnel: [w431] -> w425
                    tunnel: [w430] -> w424
                    frame #0 {
                      n243 = call <vilib>:"High Resolution Relative Seconds.vi"() -> ("relative seconds"=w430:dbl)
                    }
                  }
                  n244 = Byte Array To String(unsigned byte array=u8[] [75, 0, 4, 17, 0, 0, 0, 0] ("appended array")) -> (string=w427:string)
                  n245 = property class="VISAName"(reference=w416, error in=w429) -> (error out=w421:errorcluster, "Value"=w422:refnum<visa-resource-name>)  [unwired: 1 out]
                  n246 = VISA Write(VISA resource name=w422, write buffer=w427, error in (no error)=w421) -> (VISA resource name out=w426:refnum<visa-resource-name>, error out=w428:errorcluster)  [unwired: 1 out]
                  n247 = while {
                    tunnel: w426 -> [w445]
                    tunnel: w425 -> [w444]
                    tunnel: [w443] -> _
                    tunnel: [w442] -> w420
                    tunnel: w424 -> [w440]
                    tunnel: [w434] -> w419
                    tunnel: w417 -> [w432]
                    stop <- w436 stop-if-true
                    n248 = call <vilib>:"High Resolution Relative Seconds.vi"() -> ("relative seconds"=w441:dbl)
                    n249 = Subtract(x=w441, y=w440) -> (x-y=w439:dbl)
                    n250 = Greater Or Equal?(x=w439, y=2.0) -> (x >= y?=w437:bool)
                    n251 = property on="Stop Button" class="Bool (strict)"() -> ("Value"=w433:bool)  [unwired: 2 in, 2 out]
                    n252 = VISA Read(VISA resource name=w445, byte count=u32 1, error in (no error)=w444) -> (VISA resource name out=w447:refnum<visa-resource-name>, read buffer=w448:string, error out=w446:errorcluster)  [unwired: 1 out]
                    n253 = String To Byte Array(string=w448) -> (unsigned byte array=w451:u8[])
                    n254 = Index Array(array=w451, index=0) -> (element=w449:u8)
                    n255 = case shown="75" w449 {
                      tunnel: [w456 w461] -> w442
                      tunnel: w447 -> [w455 w470]
                      tunnel: w446 -> [w456 w469]
                      tunnel: [w455 w462] -> w443
                      tunnel: [u32 9999 w459] -> w434
                      tunnel: [FALSE w458] -> w435
                      tunnel: w432 -> [_ w457]
                      frame 0, Default {
                      }
                      frame 75 {
                        n256 = VISA Read(VISA resource name=w470, byte count=u32 3, error in (no error)=w469) -> (VISA resource name out=w465:refnum<visa-resource-name>, read buffer=w473:string, error out=w464:errorcluster)  [unwired: 1 out]
                        n257 = String To Byte Array(string=w473) -> (unsigned byte array=w463:u8[])
                        n258 = Index Array(array=w463, index #1=0 ("index")) -> (element #1=w468:u8, element #2=w466:u8)  [unwired: 2 in, 1 out]
                        n259 = Equal?(x=u8 0, y=w468) -> (x = y?=w467:bool)
                        n260 = case shown="True" w467 {
                          tunnel: [w476 w484] -> w461
                          tunnel: w466 -> [_ w491]
                          tunnel: w465 -> [w477 w490]
                          tunnel: w464 -> [w476 w489]
                          tunnel: w463 -> [_ w488]
                          tunnel: [w477 w486] -> w462
                          tunnel: [u32 9999 w480] -> w459
                          tunnel: [FALSE w479] -> w458
                          tunnel: w457 -> [_ w478]
                          frame False {
                          }
                          frame True {
                            n261 = VISA Read(VISA resource name=w490, byte count=w491, error in (no error)=w489) -> (VISA resource name out=w486:refnum<visa-resource-name>, read buffer=w485:string, error out=w484:errorcluster)  [unwired: 1 out]
                            n262 = String To Byte Array(string=w485) -> (unsigned byte array=w487:u8[])
                            n263 = Insert Into Array(array=w488, new element=w487) -> (w481:u8[])  [unwired: 1 in]
                            n264 = Index Array(array=w481, index #1=0 ("index")) -> (element #3=w482:u8)  [unwired: 2 in, 2 out]
                            n265 = case shown="15..19" w482 {
                              tunnel: w481 -> [_ w505]
                              tunnel: [u32 9999 w495] -> w480
                              tunnel: [FALSE w496] -> w479
                              tunnel: w478 -> [_ w494]
                              frame 0, Default {
                              }
                              frame 15..19 {
                                n266 = Index Array(array=w505, index #1=3 ("index")) -> (element #1=w504:u8, element #2=w503:u8, element #3=w502:u8, element #4=w501:u8)  [unwired: 3 in]
                                n267 = Join Numbers(hi=w501, lo=w502) -> ((hi.lo)=w499:u16)
                                n268 = Join Numbers(hi=w503, lo=w504) -> ((hi.lo)=w500:u16)
                                n269 = Join Numbers(hi=w499, lo=w500) -> ((hi.lo)=w497:u32)
                                n270 = Multiply(x=0.02003173828125, y=w497) -> (x*y=w495:dbl)
                                n271 = Greater Or Equal?(x=w495, y=w494) -> (x >= y?=w496:bool)
                              }
                            }
                          }
                        }
                      }
                    }
                    n272 = Compound Arithmetic op=OR(w433, w437, w435) -> (w436:bool)
                  }
                }
                n273 = Add Array Elements(numeric array=w397) -> (sum=w396:dbl)
                n274 = Divide(x=w396, y=10.0) -> (x/y=w394:dbl)
                n275 = Subtract(x=w394, y=w403) -> (x-y=w404:dbl)
                "VC15100-1 Cur" <- w404
                n276 = Greater Or Equal?(x=w404, y=w391) -> (x >= y?=w405:bool)
                n277 = And(x=w405, y=w406) -> ()  [unwired: 1 out]
              }
              frame "MD0" {
                n278 = property on="Property Node" class="Bool (strict)"(error in=w579) -> (error out=w575:errorcluster, "Value"=w581:bool)  [unwired: 1 in, 1 out]
                n279 = control-ref of="Pannel User Message"() -> (w576:refnum<vi>)
                n280 = Select(t=T8."VC15100-1", s=w581, f=T8."STOP") -> (s? t:f=w582:T8)
                n281 = property class="Str"(reference=w576, error in=w575, "Value"="7.5.2.4.Motor rotation direction test in process..." ("string")) -> (error out=w574:errorcluster)  [unwired: 1 out]
                n282 = case shown="True" w581 {
                  tunnel: [w585 w595] -> w578
                  tunnel: w574 -> [w585 w594]
                  tunnel: w573 -> [_ w589]
                  frame False {
                    n283 = call "Display Message to User"() -> ()  [unwired: 10 in, 2 out]
                  }
                  frame True {
                    (unwired) TRUE ("Remote")
                    # "Venable + Power ON"
                    # "Venable + Power OFF"
                    n284 = control-ref of="VISA resource name out"() -> (w602:refnum<vi>)
                    n285 = property on="Property Node" class="VISAName"() -> ("Value"=w615:refnum<visa-resource-name>)  [unwired: 2 in, 2 out]
                    n286 = control-ref of="Config_CANAT"() -> (w608:refnum<vi>)
                    n287 = control-ref of="UUT"() -> (w609:refnum<vi>)
                    n288 = control-ref of="Motor Speed RPM"() -> (w587:refnum<vi>)
                    n289 = control-ref of="Pannel User Message"() -> (w593:refnum<vi>)
                    n290 = Byte Array To String(unsigned byte array=u8[] [75, 0, 4, 2, 0, 0, 2, 0]) -> (string=w600:string)
                    n291 = Byte Array To String(unsigned byte array=u8[] [75, 0, 4, 2, 0, 0, 18, 0]) -> (string=w603:string)
                    n292 = VISA Flush I/O Buffer(VISA resource name=w615) -> (VISA resource name out=w616:refnum<visa-resource-name>)  [unwired: 2 in, 1 out]
                    n293 = Concatenate Strings("EP=1\r\nMD[1]=" ("write buffer"), "0" ("string"), "\r\n" ("string")) -> (w614:string)
                    n294 = call "CANSendMotorSpeed.vi"("error in (no error)"=w594, "Motor Speed RPM"=u16 0, "UUT"=w609, "Cluster in"=w608) -> ("error out"=w606:errorcluster)  [unwired: 7 in]
                    n295 = call "SerialMarvinMod.vi"("error in (no error)"=w606, "Clear Log"=FALSE, "write buffer"=w614, "VISA resource name"=w616) -> ("error out"=w605:errorcluster)  [unwired: 6 in, 1 out]
                    n296 = call <vilib>:"Clear Errors.vi"("error in (no error)"=w605) -> ("error out"=w596:errorcluster)  [unwired: 5 in, 1 out]
                    n297 = property class="VISAName"(reference=w602, error in=w596) -> (error out=w601:errorcluster, "Value"=w604:refnum<visa-resource-name>)  [unwired: 1 out]
                    n298 = VISA Write(VISA resource name=w604, write buffer=w603, error in (no error)=w601) -> (VISA resource name out=w599:refnum<visa-resource-name>, error out=w591:errorcluster)  [unwired: 1 out]
                    n299 = call "Write panel message (SubVI).vi"(4:"rpm"=w587, 5:"rpm"=FALSE ("rpm"), "Stop"=w589, "error in (no error)"=w591, "Time to wait"=15.0, "Strin"="7.5.2.4.Motor rotation direction test in process...\nSet parameters" ("string"), "String in"=w593) -> ("error out"=w590:errorcluster)  [unwired: 4 in]
                    n300 = VISA Write(VISA resource name=w599, write buffer=w600, error in (no error)=w590) -> (error out=w595:errorcluster)  [unwired: 2 out]
                  }
                }
              }
            }
            n301 = property on="Stop Button" class="Bool (strict)"() -> ("Value"=w169:bool)  [unwired: 2 in, 2 out]
            n302 = Compound Arithmetic op=OR(w171, w169) -> (w170:bool)
          }
        }
        frame Disabled {
          n303 = call "Display Message to User2"("error in (no error)"=w618) -> ("error out"=w617:errorcluster, "YES"=w619:bool)  [unwired: 9 in]
        }
      }
      n304 = And(x=w76, y=w75) -> (x .and. y?=→"EnableTestind":bool)
      n305 = call "CANSendMotorSpeed.vi"("Remote"=FALSE, "error in (no error)"=w79, "Motor Speed RPM"=u16 0, "UUT"=w81, "Cluster in"=w80) -> ("error out"=w78:errorcluster)  [unwired: 6 in]
      n306 = property class="Tbl (strict)"(reference=w53, error in=w78) -> (reference out=w112:refnum<vi>, error out=w119:errorcluster, "Value"=w118:string[][])
      n307 = Index Array(array=w118, index (col)=0 ("disabled index (col)")) -> (element=w117:string[])  [unwired: 1 in]
      n308 = call "Find_Number_LineMARVIN.vi"("Test Paragraph"="7.5.2.4", "error in"=w119, "Row Headers[]"=w117) -> ("error out"=w116:errorcluster, "Line number"=w113:i32)  [unwired: 2 in, 2 out]
      n309 = call "PassOrFail (SubVI).vi"("disabled index (col)"=6, "index (row)"=w113, "error in (no error)"=w116, "Boolean"=w75, "Table in"=w112) -> ("error out"=w114:errorcluster)  [unwired: 6 in]
      n310 = disable-structure shown="Enabled" {
        disable-tunnel: w114 -> [w146 w152]
        disable-tunnel: w113 -> [w143 _]
        disable-tunnel: _ -> [w142 _]
        disable-tunnel: w112 -> [w141 _]
        disable-tunnel: [w140 w152] -> w89
        frame Disabled {
          n311 = property class="Tbl (strict)"(reference=w141, error in=w146) -> (reference out=w151:refnum<vi>, error out=w147:errorcluster, "Value"=w150:string[][])
          n312 = Number To Fractional String(number=w142, precision (6)=i16 4) -> (F-format string=w144:string)  [unwired: 2 in]
          n313 = Replace Array Subset(array=w150, new element=w144, index (row)=w143, index (col)=5 ("disabled index (col)")) -> (w149:string[][])
          n314 = property class="Tbl (strict)"(reference=w151, error in=w147, "Value"=w149) -> (error out=w140:errorcluster)  [unwired: 1 out]
        }
        frame Enabled {
        }
      }
      n315 = property class="VISAName"(reference=w98, error in=w89) -> (error out=w97:errorcluster, "Value"=w107:refnum<visa-resource-name>)  [unwired: 1 out]
      n316 = VISA Write(VISA resource name=w107, write buffer=w99, error in (no error)=w97) -> (error out=w66:errorcluster)  [unwired: 2 out]
      n317 = call <vilib>:"Clear Errors.vi"("error in (no error)"=w66) -> ("error out"=w65:errorcluster)  [unwired: 5 in, 1 out]
      n318 = call "Time Delay2"("error in (no error)"=w65) -> ("error out"=w51:errorcluster)  [unwired: 10 in]
      n319 = property on="Property Node" class="Bool (strict)"(error in=w51, "DisabledEnum"=w68) -> (error out=w67:errorcluster)  [unwired: 1 in, 1 out]
      n320 = property on="Property Node" class="Bool (strict)"(error in=w67, "DisabledEnum"=w68) -> ()  [unwired: 1 in, 2 out]
    }
    frame "Speed Command" {
      w711 = T9."Disabled and Grayed Out" ("Disabled")
      w715 = T9."Enabled" ("Disabled")
      w795 = "7.5.3" ("Test Paragraph")
      w704 = "7.5.4" ("Test Paragraph")
      n321 = control-ref of="Pannel User Message"() -> (w726:refnum<vi>)
      n322 = property on="Property Node" class="Bool (strict)"(error in=w710, "DisabledEnum"=w711) -> (error out=w712:errorcluster)  [unwired: 1 in, 1 out]
      n323 = property class="Str"(reference=w726, error in=w710, "Value"="7.5.4.Speed Command Test") -> (error out=w725:errorcluster)  [unwired: 1 out]
      n324 = Initialize Array(FALSE, 14 ("dimension size")) -> (w773:bool[])
      n325 = property on="Property Node" class="Bool (strict)"(error in=w712, "DisabledEnum"=w711) -> ()  [unwired: 1 in, 2 out]
      n326 = Build Array (concatenate)(w773, bool[] [FALSE, FALSE, FALSE, TRUE, FALSE, FALSE, FALSE] ("array")) -> (w774:bool[])
      n327 = call "Table_ScrollaBarMarvin.vi"("error in"=w725, "Line to focus"=w704, "reference in"=w705) -> ("error out"=w806:errorcluster)  [unwired: 2 out]
      n328 = Boolean Array To Number(Boolean array=w774) -> (number=w772:u32)
      n329 = call "Reset old test Values (SubVI).vi"("error in"=w806, "Atr in"=w705, "Test Paragraph"=w704) -> ("error out"=w706:errorcluster)  [unwired: 8 in]
      n330 = property class="Tbl (strict)"(reference=w705, error in=w706) -> (error out=w808:errorcluster, "Value"=w809:string[][])  [unwired: 1 out]
      n331 = To Unsigned Long Integer(number=w772) -> (unsigned 32bit integer=w763:u32)
      n332 = control-ref of="VISA resource name out"() -> (w737:refnum<vi>)
      n333 = control-ref of="VISA resource name out"() -> (w761:refnum<vi>)
      n334 = property on="Property Node" class="Str"() -> ("Value"=w709:string)  [unwired: 2 in, 2 out]
      n335 = control-ref of="Config_CANAT"() -> (w803:refnum<vi>)
      n336 = control-ref of="UUT"() -> (w802:refnum<vi>)
      n337 = Equal?(x=w709, y="EBAY") -> (x = y?=w707:bool)
      n338 = case shown="False" w707 {
        tunnel: [u16[] [6000, 9000, 12100] u16[] [6000, 11500, 15100]] -> w804
        frame False {
        }
        frame True {
        }
      }
      n339 = Initialize Array(FALSE, 14 ("dimension size")) -> (w749:bool[])
      n340 = Build Array (concatenate)(w749, bool[] [FALSE, FALSE, FALSE, FALSE, FALSE, FALSE, FALSE] ("array")) -> (w750:bool[])
      n341 = Boolean Array To Number(Boolean array=w750) -> (number=w748:u32)
      n342 = To Unsigned Long Integer(number=w748) -> (unsigned 32bit integer=w739:u32)
      n343 = Split Number(x=w739) -> (hi(x)=w744:u16, lo(x)=w745:u16)
      n344 = Split Number(x=w745) -> (hi(x)=w743:u8, lo(x)=w742:u8)
      n345 = flat-sequence {
        tunnel: [w814] -> w799
        tunnel: w798 -> [w813]
        tunnel: [w813] -> w797
        frame #0 {
          n346 = call <vilib>:"High Resolution Relative Seconds.vi"() -> ("relative seconds"=w814:dbl)
        }
      }
      n347 = Split Number(x=w763) -> (hi(x)=w768:u16, lo(x)=w769:u16)
      n348 = Split Number(x=w744) -> (hi(x)=w741:u8, lo(x)=w740:u8)
      n349 = Build Array(u8 75, u8 0 ("element"), u8 4 ("Length"), u8 2, w742, w743, w740, w741) -> (w747:u8[])
      n350 = Byte Array To String(unsigned byte array=w747) -> (string=w738:string)
      n351 = Split Number(x=w769) -> (hi(x)=w767:u8, lo(x)=w766:u8)
      n352 = Concatenate Strings("7.5.3.Stop Time Test in process... ", "\r\n", "Motor Speed [rpm]: " ("string")) -> (w720:string)
      n353 = while {
        tunnel: w799 -> [w830]
        tunnel: w797 -> [w824]
        tunnel: [w825] -> w776
        tunnel: [w821] -> w788
        tunnel: w720 -> [w818]
        stop <- w828 stop-if-true
        n354 = control-ref of="Motor Speed RPM"() -> (w833:refnum<vi>)
        n355 = control-ref of="Pannel User Message"() -> (w823:refnum<vi>)
        n356 = call <vilib>:"High Resolution Relative Seconds.vi"() -> ("relative seconds"=w831:dbl)
        n357 = Subtract(x=w831, y=w830) -> (x-y=w825:dbl)
        n358 = property class="DigNum (strict)"(reference=w833, error in=w824) -> (error out=w822:errorcluster, "Value"=w816:dbl)  [unwired: 1 out]
        n359 = Number To Fractional String(number=w816, precision (6)=i16 2) -> (F-format string=w817:string)  [unwired: 2 in]
        n360 = Concatenate Strings(w818, w817) -> (w819:string)
        n361 = property class="Str"(reference=w823, error in=w822, "Value"=w819) -> (error out=w821:errorcluster)  [unwired: 1 out]
        n362 = Less Or Equal?(x=w816, y=0.0) -> (x <= y?=w827:bool)
        n363 = Greater Or Equal?(x=w825, y=50.0) -> (x >= y?=w826:bool)
        n364 = property on="Stop Button" class="Bool (strict)"() -> ("Value"=w815:bool)  [unwired: 2 in, 2 out]
        n365 = Compound Arithmetic op=OR(w827, w826, w815) -> (w828:bool)
      }
      n366 = Less?(x=w776, y=50.0) -> (x < y?=w718:bool)
      n367 = call "Table_ScrollaBarMarvin.vi"("error in"=w788, "Line to focus"=w795, "reference in"=w705) -> ("error out"=w796:errorcluster)  [unwired: 2 out]
      n368 = property class="Tbl (strict)"(reference=w705, error in=w796) -> (reference out=w775:refnum<vi>, error out=w793:errorcluster, "Value"=w792:string[][])
      n369 = Index Array(array=w792, index (col)=0 ("disabled index (col)")) -> (element=w791:string[])  [unwired: 1 in]
      n370 = call "Find_Number_LineMARVIN.vi"("Test Paragraph"=w795, "error in"=w793, "Row Headers[]"=w791) -> ("error out"=w789:errorcluster, "Line number"=w790:i32)  [unwired: 2 in, 2 out]
      n371 = Increment(x=w790) -> (x+1=w777:i32)
      n372 = call "PassOrFail (SubVI).vi"("disabled index (col)"=6, "index (row)"=w777, "error in (no error)"=w789, "Boolean"=w718, "Table in"=w775) -> ("error out"=w781:errorcluster)  [unwired: 6 in]
      n373 = property class="Tbl (strict)"(reference=w775, error in=w781) -> (reference out=w786:refnum<vi>, error out=w782:errorcluster, "Value"=w785:string[][])
      n374 = Index Array(array=w809, index (col)=0 ("disabled index (col)")) -> (element=w810:string[])  [unwired: 1 in]
      n375 = Number To Fractional String(number=w776, precision (6)=i16 2) -> (F-format string=w778:string)  [unwired: 2 in]
      n376 = Replace Array Subset(array=w785, new element=w778, index (row)=w777, index (col)=5 ("disabled index (col)")) -> (w784:string[][])
      n377 = property class="Tbl (strict)"(reference=w786, error in=w782, "Value"=w784) -> (error out=w728:errorcluster)  [unwired: 1 out]
      n378 = property class="VISAName"(reference=w737, error in=w728) -> (error out=w736:errorcluster, "Value"=w746:refnum<visa-resource-name>)  [unwired: 1 out]
      n379 = VISA Write(VISA resource name=w746, write buffer=w738, error in (no error)=w736) -> (error out=w713:errorcluster)  [unwired: 2 out]
      n380 = property on="Property Node" class="Bool (strict)"(error in=w713, "DisabledEnum"=w715) -> (error out=w714:errorcluster)  [unwired: 1 in, 1 out]
      n381 = property on="Property Node" class="Bool (strict)"(error in=w714, "DisabledEnum"=w715) -> ()  [unwired: 1 in, 2 out]
      n382 = Split Number(x=w768) -> (hi(x)=w765:u8, lo(x)=w764:u8)
      n383 = Build Array(u8 75, u8 0 ("element"), u8 4 ("Length"), u8 2, w766, w767, w764, w765) -> (w771:u8[])
      n384 = Byte Array To String(unsigned byte array=w771) -> (string=w762:string)
      n385 = call "Find_Number_LineMARVIN.vi"("Test Paragraph"=w704, "error in"=w808, "Row Headers[]"=w810) -> ("error out"=w752:errorcluster, "Line number"=w805:i32)  [unwired: 2 in, 2 out]
      n386 = property class="VISAName"(reference=w761, error in=w752) -> (error out=w760:errorcluster, "Value"=w770:refnum<visa-resource-name>)  [unwired: 1 out]
      n387 = VISA Write(VISA resource name=w770, write buffer=w762, error in (no error)=w760) -> (error out=w751:errorcluster)  [unwired: 2 out]
      n388 = for {
        tunnel: w751 -> [w858]
        tunnel: w705 -> [w855]
        tunnel: w805 -> [w844]
        tunnel: w804 -> [w847] mode=indexing
        tunnel: [w842] -> w801
        tunnel: [w834] -> w719 mode=indexing
        i -> [w846]
        w848 = 200.0 ("y")
        n389 = control-ref of="Config_CANAT"() -> (w864:refnum<vi>)
        n390 = control-ref of="Motor Speed RPM"() -> (w863:refnum<vi>)
        n391 = control-ref of="UUT"() -> (w865:refnum<vi>)
        n392 = Add(x=w847, y=w848) -> (x+y=w850:dbl)
        n393 = Subtract(x=w847, y=w848) -> (x-y=w849:dbl)
        n394 = Increment(x=w846) -> (x+1=w845:i32)
        n395 = Add(x=w844, y=w845) -> (x+y=w841:i32)
        n396 = call "CANSendMotorSpeed.vi"("Remote"=TRUE, "error in (no error)"=w858, "Motor Speed RPM"=w847, "UUT"=w865, "Cluster in"=w864) -> ("error out"=w839:errorcluster)  [unwired: 6 in]
        n397 = call <vilib>:"High Resolution Relative Seconds.vi"() -> ("relative seconds"=w835:dbl)
        n398 = while {
          tunnel: w839 -> [w885]
          tunnel: [w885] -> w838
          tunnel: "7.5.4.Speed Command Test" ("Value") -> [w882]
          tunnel: "Time to wait: " ("Value") -> [w880]
          tunnel: w835 -> [w878]
          stop <- w870 stop-if-true
          n399 = control-ref of="Pannel User Message"() -> (w884:refnum<vi>)
          n400 = call <vilib>:"High Resolution Relative Seconds.vi"() -> ("relative seconds"=w879:dbl)
          n401 = Subtract(x=w879, y=w878) -> (x-y=w876:dbl)
          n402 = property on="Stop Button" class="Bool (strict)"() -> ("Value"=w869:bool)  [unwired: 2 in, 2 out]
          n403 = Subtract(x=35.0, y=w876) -> (x-y=w871:dbl)
          n404 = Less Or Equal To 0?(x=w871) -> (x <= 0?=w877:bool)
          n405 = Compound Arithmetic op=OR(w877, w869) -> (w870:bool)
          n406 = Number To Fractional String(number=w871, precision (6)=i16 2) -> (F-format string=w873:string)  [unwired: 2 in]
          n407 = property on="Motor Speed RPM" class="DigNum (strict)"() -> ("Value"=w867:dbl)  [unwired: 2 in, 2 out]
          n408 = Number To Fractional String(number=w867, precision (6)=i16 2) -> (F-format string=w866:string)  [unwired: 2 in]
          n409 = Concatenate Strings(w882, "\r\n", w880, w873, "  Sec.\nMotor speed [rpm]: " ("string"), w866) -> (w883:string)
          n410 = property class="Str"(reference=w884, "Value"=w883) -> ()  [unwired: 1 in, 2 out]
        }
        n411 = property class="DigNum (strict)"(reference=w863, error in=w838) -> (error out=w856:errorcluster, "Value"=w857:dbl)  [unwired: 1 out]
        n412 = In Range and Coerce(upper limit=w850, x=w857, lower limit=w849) -> (In Range?=w834:bool)  [unwired: 1 out]
        n413 = call "PassOrFail (SubVI).vi"("disabled index (col)"=6, "index (row)"=w841, "error in (no error)"=w856, "Boolean"=w834, "Table in"=w855) -> ("error out"=w860:errorcluster)  [unwired: 6 in]
        n414 = property class="Tbl (strict)"(reference=w855, error in=w860) -> (reference out=w851:refnum<vi>, error out=w861:errorcluster, "Value"=w852:string[][])
        n415 = Number To Fractional String(number=w857, precision (6)=i16 2) -> (F-format string=w854:string)  [unwired: 2 in]
        n416 = Replace Array Subset(array=w852, new element=w854, index (row)=w841, index (col)=5 ("disabled index (col)")) -> (w853:string[][])
        n417 = property class="Tbl (strict)"(reference=w851, error in=w861, "Value"=w853) -> (error out=w842:errorcluster)  [unwired: 1 out]
      }
      n418 = call "CANSendMotorSpeed.vi"("Remote"=TRUE, "error in (no error)"=w801, "Motor Speed RPM"=u16 0, "UUT"=w802, "Cluster in"=w803) -> ("error out"=w798:errorcluster)  [unwired: 6 in]
      n419 = Build Array (concatenate)(w719, w718) -> (w717:bool[])
      n420 = And Array Elements(Boolean array=w717) -> (logical AND=→"SpeedStopind":bool)
    }
    frame "Stop Time" {
      w903 = T9."Enabled" ("Disabled")
      w904 = T9."Disabled and Grayed Out" ("Disabled")
      w891 = "9.Motor Temperature  test in process..." ("Value")
      w900 = "9" ("Test Paragraph")
      # "k15 = 64\nk16 = 128"
      # "K15+Venable"
      # "Deg"
      # "K15 OFF"
      n421 = property on="Stop Button" class="Bool (strict)"("DisabledEnum"=w904) -> ()  [unwired: 2 in, 2 out]
      n422 = property on="Property Node" class="Bool (strict)"(error in=w908, "DisabledEnum"=w904) -> (error out=w909:errorcluster)  [unwired: 1 in, 1 out]
      n423 = Byte Array To String(unsigned byte array=u8[] [75, 0, 4, 2, 0, 64, 0, 0] ("appended array")) -> ()  [unwired: 1 out]
      n424 = property on="Property Node" class="Bool (strict)"(error in=w909, "DisabledEnum"=w904) -> (error out=w907:errorcluster)  [unwired: 1 in, 1 out]
      n425 = control-ref of="VISA resource name out"() -> (w929:refnum<vi>)
      n426 = control-ref of="Stop Button"() -> (w894:refnum<vi>)
      n427 = control-ref of="Config_CANAT"() -> (w920:refnum<vi>)
      n428 = control-ref of="UUT"() -> (w921:refnum<vi>)
      n429 = control-ref of="Motor Speed RPM"() -> (w892:refnum<vi>)
      n430 = control-ref of="Pannel User Message"() -> (w925:refnum<vi>)
      n431 = control-ref of="Pannel User Message"() -> (w893:refnum<vi>)
      n432 = Byte Array To String(unsigned byte array=u8[] [75, 0, 4, 2, 0, 0, 0, 0] ("appended array")) -> (string=w932:string)
      n433 = property on="Index" class="Str"() -> ("Value"=w890:string)  [unwired: 2 in, 2 out]
      n434 = Decimal String To Number(string=w890) -> (number=w889:i32)  [unwired: 2 in, 1 out]
      n435 = Subtract(x=w889, y=3 ("x")) -> (x-y=w888:i32)
      n436 = Number To Decimal String(number=w888) -> (decimal integer string=w887:string)  [unwired: 1 in]
      n437 = property class="Str"(reference=w925, error in=w907, "Value"=w891) -> (error out=w924:errorcluster)  [unwired: 1 out]
      n438 = call "Reset old test Values (SubVI).vi"("error in"=w924, "Atr in"=w901, "Test Paragraph"=w900) -> ("error out"=w902:errorcluster)  [unwired: 8 in]
      n439 = call "Table_ScrollaBarMarvin.vi"("error in"=w902, "Line to focus"=w900, "reference in"=w901) -> ("error out"=w939:errorcluster)  [unwired: 2 out]
      n440 = property class="Tbl (strict)"(reference=w901, error in=w939) -> (reference out=w923:refnum<vi>, error out=w938:errorcluster, "Value"=w937:string[][])
      n441 = Index Array(array=w937, index (col)=0 ("disabled index (col)")) -> (element=w936:string[])  [unwired: 1 in]
      n442 = call "Find_Number_LineMARVIN.vi"("Test Paragraph"=w900, "error in"=w938, "Row Headers[]"=w936) -> ("error out"=w934:errorcluster, "Line number"=w914:i32)  [unwired: 2 in, 2 out]
      n443 = call "Table_ScrollaBarMarvin.vi"("error in"=w934, "Line to focus"=w900, "reference in"=w923) -> ("error out"=w917:errorcluster)  [unwired: 2 out]
      n444 = call "CANSendMotorSpeed.vi"("Remote"=FALSE, "error in (no error)"=w917, "Motor Speed RPM"=u16 0, "UUT"=w921, "Cluster in"=w920) -> ("error out"=w916:errorcluster)  [unwired: 6 in]
      n445 = property class="VISAName"(reference=w929, error in=w916) -> (error out=w915:errorcluster, "Value"=w940:refnum<visa-resource-name>)  [unwired: 1 out]
      n446 = call "Write panel message (SubVI).vi"("rpm"=w892, "Stop"=w894, "error in (no error)"=w915, "Time to wait"=5.0 ("Delay Time (sec)"), "Strin"=w891, "String in"=w893) -> ("error out"=w927:errorcluster)  [unwired: 5 in]
      n447 = call "Time Delay4"("error in (no error)"=w927) -> ("error out"=w898:errorcluster)  [unwired: 10 in]
      n448 = call "Write panel message (SubVI).vi"("rpm"=w892, "PrintTime"=FALSE, "Stop"=w894, "error in (no error)"=w898, "Time to wait"=0.01, "Strin"=w891, "String in"=w893) -> ("error out"=w897:errorcluster)  [unwired: 4 in]
      n449 = call <vilib>:"Clear Errors.vi"("error in (no error)"=w897) -> ("error out"=w899:errorcluster)  [unwired: 5 in, 1 out]
      n450 = for {
        tunnel: w899 -> [w991]
        tunnel: dbl[] [1288.0, 1569.0, 1774.0] -> [w971] mode=indexing
        tunnel: w923 -> [w985]
        tunnel: w923 -> [w980]
        tunnel: [w973] -> w905
        tunnel: w940 -> [w979]
        tunnel: w914 -> [w969]
        tunnel: dbl[] [60.0, 90.0, 110.0] -> [w966] mode=indexing
        tunnel: [w964] -> w912 mode=indexing
        tunnel: u32[] [128, 1024, 4096] -> [w950] mode=indexing
        tunnel: w894 -> [w947]
        tunnel: w893 -> [w946]
        tunnel: w892 -> [w945]
        tunnel: w891 -> [w942]
        tunnel: w887 -> [w941]
        i -> [w963]
        w972 = 3.0 ("y")
        n451 = Add(x=w966, y=w972) -> (x+y=w976:dbl)
        n452 = Increment(x=w969) -> (x+1=w968:i32)
        n453 = Subtract(x=w966, y=w972) -> (x-y=w977:dbl)
        n454 = Add(x=w968, y=w963) -> (x+y=w967:i32)
        n455 = call "DegToDAC (SubVI).vi"("error in (no error)"=w991, "R2"=10.0, "Numeric"=w971) -> ("error out"=w975:errorcluster)  [unwired: 7 in, 1 out]
        n456 = To Unsigned Long Integer(number=w950) -> (unsigned 32bit integer=w953:u32)
        n457 = Split Number(x=w953) -> (hi(x)=w958:u16, lo(x)=w959:u16)
        n458 = Split Number(x=w959) -> (hi(x)=w957:u8, lo(x)=w956:u8)
        n459 = Split Number(x=w958) -> (hi(x)=w955:u8, lo(x)=w954:u8)
        n460 = Build Array(u8 75, u8 0 ("element"), u8 4 ("Length"), u8 2, w956, w957, w954, w955) -> (w951:u8[])
        n461 = Byte Array To String(unsigned byte array=w951) -> (string=w949:string)
        n462 = VISA Write(VISA resource name=w979, write buffer=w949, error in (no error)=w975) -> (error out=w978:errorcluster)  [unwired: 2 out]
        n463 = call "Write panel message (SubVI).vi"(4:"rpm"=w945, 5:"rpm"=FALSE ("rpm"), "PrintTime"=TRUE, "Stop"=w947, "error in (no error)"=w978, "Time to wait"=3.0, "Strin"=w942, "String in"=w946) -> ("error out"=w970:errorcluster)  [unwired: 3 in]
        n464 = disable-structure shown="Enabled" {
          disable-tunnel: [w995 w1005] -> w984
          disable-tunnel: [w993 w1001] -> w974
          disable-tunnel: w970 -> [w992 w1004]
          disable-tunnel: w941 -> [_ w996]
          frame Disabled {
            n465 = control-ref of="Motor Stator Temp."() -> (w994:refnum<vi>)
            n466 = property class="DigNum (strict)"(reference=w994, error in=w992) -> (error out=w995:errorcluster, "Value"=w993:dbl)  [unwired: 1 out]
          }
          frame Enabled {
            n467 = for {
              N: 6 -> [_]
              tunnel: [w1018] -> w1006 mode=indexing
              tunnel: w1004 -> [w1014]
              tunnel: [w1017] -> w1005
              tunnel: w996 -> [w1008]
              n468 = property on="Property Node" class="VISAName"() -> ("Value"=w1015:refnum<visa-resource-name>)  [unwired: 2 in, 2 out]
              n469 = Search and Replace String(input string="TA[2]\r\n" ("write buffer"), search string="2", replace string=w1008) -> (result string=w1007:string)  [unwired: 5 in, 3 out]
              n470 = call "Time Delay3"("error in (no error)"=w1014) -> ("error out"=w1011:errorcluster)  [unwired: 10 in]
              n471 = VISA Flush I/O Buffer(VISA resource name=w1015, error in (no error)=w1011) -> (VISA resource name out=w1012:refnum<visa-resource-name>, error out=w1013:errorcluster)  [unwired: 1 in]
              n472 = call "SerialMarvinMod.vi"("error in (no error)"=w1013, "write buffer"=w1007, "VISA resource name"=w1012) -> ("error out"=w1017:errorcluster, "read buffer"=w1016:string)  [unwired: 7 in]
              n473 = Fract/Exp String To Number(string=w1016) -> (number=w1018:dbl)  [unwired: 3 in, 1 out]
            }
            n474 = Delete From Array(array=w1006, length=1, index=0) -> (array with subset deleted=w999:dbl[])  [unwired: 1 out]
            n475 = Add Array Elements(numeric array=w999) -> (sum=w1002:dbl)
            n476 = Divide(x=w1002, y=5.0) -> (x/y=w1001:dbl)
          }
        }
        n477 = In Range and Coerce(upper limit=w976, x=w974, lower limit=w977) -> (In Range?=w964:bool)  [unwired: 1 out]
        n478 = call "PassOrFail (SubVI).vi"("disabled index (col)"=6, "index (row)"=w967, "error in (no error)"=w984, "Boolean"=w964, "Table in"=w980) -> ("error out"=w988:errorcluster)  [unwired: 6 in]
        n479 = property class="Tbl (strict)"(reference=w985, error in=w988) -> (error out=w981:errorcluster, "Value"=w990:string[][])  [unwired: 1 out]
        n480 = Number To Fractional String(number=w974, precision (6)=i16 2) -> (F-format string=w989:string)  [unwired: 2 in]
        n481 = Replace Array Subset(array=w990, new element=w989, index (row)=w967, index (col)=5 ("disabled index (col)")) -> (w982:string[][])
        n482 = property class="Tbl (strict)"(reference=w980, error in=w981, "Value"=w982) -> (error out=w973:errorcluster)  [unwired: 1 out]
      }
      n483 = property on="Property Node" class="Bool (strict)"(error in=w905, "DisabledEnum"=w903) -> (error out=w906:errorcluster)  [unwired: 1 in, 1 out]
      n484 = property on="Property Node" class="Bool (strict)"(error in=w906, "DisabledEnum"=w903) -> ()  [unwired: 1 in, 2 out]
      n485 = And Array Elements(Boolean array=w912) -> (logical AND=→"MotorTempind":bool)
      n486 = property class="VISAName"(reference=w929, error in=w905) -> (error out=w931:errorcluster, "Value"=w933:refnum<visa-resource-name>)  [unwired: 1 out]
      n487 = VISA Write(VISA resource name=w933, write buffer=w932, error in (no error)=w931) -> ()  [unwired: 3 out]
      n488 = property on="Stop Button" class="Bool (strict)"("DisabledEnum"=w903) -> ()  [unwired: 2 in, 2 out]
    }
    frame "Temp Control" {
      (unwired) dbl[] [5927.0, 11480.0, 15061.0, 11530.0, 6175.0]
      w1034 = T9."Enabled" ("Disabled")
      w1036 = T9."Disabled and Grayed Out" ("Disabled")
      w1019 = "7.5.6" ("Test Paragraph")
      # "K16+Venable"
      # "Deg"
      # "K16 OFF + Venable"
      # "Venable"
      n489 = flat-sequence {
        tunnel: w1032 -> [_]
        frame #0 {
          "TempAlg" <- TRUE
        }
      }
      n490 = control-ref of="Pannel User Message"() -> (w1058:refnum<vi>)
      n491 = property class="Str"(reference=w1058, error in=w1032, "Value"="7.5.6.Temperature controle test") -> (error out=w1057:errorcluster)  [unwired: 1 out]
      n492 = property on="Property Node" class="Bool (strict)"(error in=w1032, "DisabledEnum"=w1036) -> (error out=w1037:errorcluster)  [unwired: 1 in, 1 out]
      n493 = call "Reset old test Values (SubVI).vi"("error in"=w1057, "Atr in"=w1020, "Test Paragraph"=w1019) -> ("error out"=w1021:errorcluster)  [unwired: 8 in]
      n494 = property on="Property Node" class="Bool (strict)"(error in=w1037, "DisabledEnum"=w1036) -> ()  [unwired: 1 in, 2 out]
      n495 = call "Table_ScrollaBarMarvin.vi"("error in"=w1021, "Line to focus"=w1019, "reference in"=w1020) -> ("error out"=w1078:errorcluster)  [unwired: 2 out]
      n496 = property class="Tbl (strict)"(reference=w1020, error in=w1078) -> (reference out=w1055:refnum<vi>, error out=w1077:errorcluster, "Value"=w1076:string[][])
      n497 = control-ref of="VISA resource name out"() -> (w1068:refnum<vi>)
      n498 = control-ref of="Config_CANAT"() -> (w1049:refnum<vi>)
      n499 = control-ref of="UUT"() -> (w1050:refnum<vi>)
      n500 = Byte Array To String(unsigned byte array=u8[] [75, 0, 4, 2, 0, 0, 0, 0] ("appended array")) -> (string=w1070:string)
      n501 = while {
        tunnel: [w1102] -> w1028
        stop <- w1103 stop-if-true
        w1105 = 6050.0 ("y")
        n502 = Random Number (0-1)() -> (number: 0 to 1=w1106:dbl)
        n503 = Multiply(x=w1106, y=w1105) -> (x*y=w1102:dbl)
        n504 = In Range and Coerce(upper limit=w1105, x=w1102, lower limit=5950.0) -> (In Range?=w1103:bool)  [unwired: 1 out]
      }
      n505 = Index Array(array=w1076, index (col)=0 ("disabled index (col)")) -> (element=w1075:string[])  [unwired: 1 in]
      n506 = while {
        tunnel: [w1087] -> w1027
        stop <- w1088 stop-if-true
        w1090 = 11550.0 ("y")
        n507 = Random Number (0-1)() -> (number: 0 to 1=w1091:dbl)
        n508 = Multiply(x=w1091, y=w1090) -> (x*y=w1087:dbl)
        n509 = In Range and Coerce(upper limit=w1090, x=w1087, lower limit=11450.0) -> (In Range?=w1088:bool)  [unwired: 1 out]
      }
      n510 = while {
        tunnel: [w1097] -> w1026
        stop <- w1098 stop-if-true
        w1100 = 15050.0 ("y")
        n511 = Random Number (0-1)() -> (number: 0 to 1=w1101:dbl)
        n512 = Multiply(x=w1101, y=w1100) -> (x*y=w1097:dbl)
        n513 = In Range and Coerce(upper limit=w1100, x=w1097, lower limit=14950.0) -> (In Range?=w1098:bool)  [unwired: 1 out]
      }
      n514 = while {
        tunnel: [w1092] -> w1025
        stop <- w1093 stop-if-true
        w1095 = 11550.0 ("y")
        n515 = Random Number (0-1)() -> (number: 0 to 1=w1096:dbl)
        n516 = Multiply(x=w1096, y=w1095) -> (x*y=w1092:dbl)
        n517 = In Range and Coerce(upper limit=w1095, x=w1092, lower limit=11450.0) -> (In Range?=w1093:bool)  [unwired: 1 out]
      }
      n518 = while {
        tunnel: [w1082] -> w1024
        stop <- w1083 stop-if-true
        w1085 = 6050.0 ("y")
        n519 = Random Number (0-1)() -> (number: 0 to 1=w1086:dbl)
        n520 = Multiply(x=w1086, y=w1085) -> (x*y=w1082:dbl)
        n521 = In Range and Coerce(upper limit=w1085, x=w1082, lower limit=5950.0) -> (In Range?=w1083:bool)  [unwired: 1 out]
      }
      n522 = Build Array(w1028, w1027, w1026, w1025, w1024) -> (w1023:dbl[])
      n523 = To Unsigned Word Integer(number=w1023) -> (unsigned 16bit integer=w1022:u16[])
      n524 = Byte Array To String(unsigned byte array=u8[] [75, 0, 4, 2, 0, 0, 2, 0] ("appended array")) -> (string=w1080:string)
      n525 = Byte Array To String(unsigned byte array=u8[] [75, 0, 4, 2, 0, 128, 2, 0] ("appended array")) -> (string=w1062:string)
      n526 = call "Find_Number_LineMARVIN.vi"("Test Paragraph"=w1019, "error in"=w1077, "Row Headers[]"=w1075) -> ("error out"=w1073:errorcluster, "Line number"=w1065:i32)  [unwired: 2 in, 2 out]
      n527 = call "Table_ScrollaBarMarvin.vi"("error in"=w1073, "Line to focus"=w1019, "reference in"=w1055) -> ("error out"=w1045:errorcluster)  [unwired: 2 out]
      n528 = call "CANSendMotorSpeed.vi"("Remote"=FALSE, "error in (no error)"=w1045, "Motor Speed RPM"=u16 0, "UUT"=w1050, "Cluster in"=w1049) -> ("error out"=w1044:errorcluster)  [unwired: 6 in]
      n529 = property class="VISAName"(reference=w1068, error in=w1044) -> (error out=w1081:errorcluster, "Value"=w1079:refnum<visa-resource-name>)  [unwired: 1 out]
      n530 = VISA Write(VISA resource name=w1079, write buffer=w1080, error in (no error)=w1081) -> (VISA resource name out=w1063:refnum<visa-resource-name>, error out=w1064:errorcluster)  [unwired: 1 out]
      n531 = call "Wait_Sec.vi"("Delay Time (sec)"=2.0, "error out"=w1064) -> ("error in"=w1060:errorcluster)  [unwired: 2 in]
      n532 = VISA Write(VISA resource name=w1063, write buffer=w1062, error in (no error)=w1060) -> (VISA resource name out=w1053:refnum<visa-resource-name>, error out=w1061:errorcluster)  [unwired: 1 out]
      n533 = call "Time Delay5"("error in (no error)"=w1061) -> ("error out"=w1046:errorcluster)  [unwired: 10 in]
      n534 = for {
        tunnel: w1046 -> [w1149]
        tunnel: dbl[] [1202.0, 1288.0, 1472.0, 1472.0, 1379.0] -> [w1118] mode=indexing
        tunnel: dbl[] [200.0, 200.0, 400.0, 200.0, 200.0] -> [w1148] mode=indexing
        tunnel: w1065 -> [w1146]
        tunnel: w1055 -> [w1139]
        tunnel: w1055 -> [w1124]
        tunnel: [w1138] -> w1054
        tunnel: w1053 -> [w1119]
        tunnel: dbl[] [6000.0, 7000.0, 12200.0, 14500.0, 11100.0] -> [w1110] mode=indexing
        tunnel: dbl[] [50.0, 68.0, 88.0, 80.0, 60.0] -> [w1117] mode=indexing
        tunnel: dbl[] [6000.0, 11400.0, 14900.0, 11600.0, 6200.0] -> [w1115] mode=indexing
        tunnel: [w1112] -> w1041 mode=indexing
        tunnel: [w1111] -> w1040 mode=indexing
        tunnel: w1022 -> [w1109] mode=indexing
        tunnel: dbl[] [57.0, 67.0, 89.0, 79.0, 61.0] -> [w1108] mode=indexing
        i -> [w1114]
        w1130 = 6 ("disabled index (col)")
        n535 = disable-structure shown="Enabled" {
          disable-tunnel: w1149 -> [w1167 w1337]
          disable-tunnel: w1148 -> [w1166 _]
          disable-tunnel: [w1165 w1335] -> w1128
          disable-tunnel: w1119 -> [w1163 _]
          disable-tunnel: w1118 -> [w1162 _]
          disable-tunnel: w1117 -> [w1161 _]
          disable-tunnel: [w1159 w1337] -> w1116
          disable-tunnel: w1115 -> [w1158 _]
          disable-tunnel: w1114 -> [w1157 _]
          disable-tunnel: [w1155 w1336] -> w1113
          disable-tunnel: [w1154 w1338] -> w1112
          disable-tunnel: [w1153 w1338] -> w1111
          disable-tunnel: w1110 -> [w1150 _]
          disable-tunnel: w1109 -> [_ w1336]
          disable-tunnel: w1108 -> [_ w1335]
          frame Enabled {
            n536 = call <vilib>:"High Resolution Relative Seconds.vi"() -> ("relative seconds"=w1164:dbl)
            n537 = while {
              tunnel: w1166 -> [w1246]
              tunnel: w1167 -> [w1258]
              tunnel: [w1241] -> w1151
              tunnel: [w1226] -> w1156
              tunnel: [w1244] -> w1154
              tunnel: [w1234] -> w1165
              tunnel: [w1233] -> w1153
              tunnel: w1157 -> [w1235]
              tunnel: w1164 -> [w1253]
              tunnel: w1163 -> [w1249]
              tunnel: w1150 -> [w1247]
              shift-right: [w1248] -> _
              shift-left: w1162 -> [w1232]
              tunnel: w1161 -> [w1231]
              shift-right: [w1223] -> _
              shift-left: "" -> [w1230]
              tunnel: [w1221] -> w1152
              stop <- w1255 stop-if-true
              n538 = control-ref of="Motor Speed RPM"() -> (w1257:refnum<vi>)
              n539 = control-ref of="Ambient Temperature"() -> (w1259:refnum<vi>)
              n540 = call <vilib>:"High Resolution Relative Seconds.vi"() -> ("relative seconds"=w1250:dbl)
              n541 = case shown="0, 1, Default" w1235 {
                tunnel: w1258 -> [w1307 w1314]
                tunnel: [w1307 w1313] -> w1229
                tunnel: w1249 -> [_ w1312]
                tunnel: w1232 -> [_ w1311]
                tunnel: [TRUE FALSE] -> w1245
                frame 10 {
                }
                frame 0, 1, Default {
                  n542 = call "DegToDAC (SubVI).vi"("error in (no error)"=w1314, "R2"=0.0, "Numeric"=w1311) -> ("error out"=w1315:errorcluster, "output array"=w1310:u8[])  [unwired: 7 in]
                  n543 = Byte Array To String(unsigned byte array=w1310) -> (string=w1316:string)
                  n544 = VISA Write(VISA resource name=w1312, write buffer=w1316, error in (no error)=w1315) -> (error out=w1313:errorcluster)  [unwired: 2 out]
                }
              }
              n545 = property class="DigNum (strict)"(reference=w1259, error in=w1229) -> (error out=w1256:errorcluster, "Value"=w1234:dbl)  [unwired: 1 out]
              n546 = case shown="1, 2" w1235 {
                tunnel: w1234 -> [w1266 w1272 w1275]
                tunnel: [w1267 w1273 w1276] -> w1233
                tunnel: w1231 -> [w1265 w1268 _]
                frame 3, 4 {
                  w1264 = 2.0 ("y")
                  n547 = Add(x=w1264, y=w1265) -> (x+y=w1263:dbl)
                  n548 = Subtract(x=w1265, y=w1264) -> (x-y=w1262:dbl)
                  n549 = In Range and Coerce(upper limit=w1263, x=w1266, lower limit=w1262) -> (In Range?=w1267:bool)  [unwired: 1 out]
                }
                frame 1, 2 {
                  w1271 = 2.0 ("y")
                  n550 = Add(x=w1271, y=w1268) -> (x+y=w1270:dbl)
                  n551 = Subtract(x=w1268, y=w1271) -> (x-y=w1269:dbl)
                  n552 = In Range and Coerce(upper limit=w1270, x=w1272, lower limit=w1269) -> (In Range?=w1273:bool)  [unwired: 1 out]
                }
                frame Default {
                  n553 = Less Or Equal?(x=w1275, y=65.0) -> (x <= y?=w1276:bool)
                }
              }
              n554 = property class="DigNum (strict)"(reference=w1257, error in=w1256) -> (error out=w1228:errorcluster, "Value"=w1241:dbl)  [unwired: 1 out]
              n555 = case shown="3, 4" w1235 {
                tunnel: [w1282 w1299] -> w1244
                tunnel: [w1286 w1303] -> w1248
                tunnel: w1232 -> [w1285 w1302]
                tunnel: w1241 -> [w1280 w1294]
                tunnel: w1247 -> [w1279 w1298]
                tunnel: w1246 -> [w1284 w1301]
                tunnel: w1228 -> [w1278 w1292]
                tunnel: [w1278 w1292] -> w1227
                frame 0, 1, Default {
                  n556 = Add(x=10.0, y=w1285) -> (x+y=w1286:dbl)
                  n557 = Greater Or Equal?(x=w1280, y=w1279) -> (x >= y?=w1281:bool)
                  n558 = Add(x=w1279, y=w1284) -> (x+y=w1287:dbl)
                  n559 = Subtract(x=w1279, y=w1284) -> (x-y=w1288:dbl)
                  n560 = In Range and Coerce(upper limit=w1287, x=w1280, lower limit=w1288) -> (In Range?=w1277:bool)  [unwired: 1 out]
                  n561 = Compound Arithmetic op=OR(w1281, w1277) -> (w1282:bool)
                }
                frame 3, 4 {
                  n562 = Subtract(x=w1302, y=10.0 ("x")) -> (x-y=w1303:dbl)
                  n563 = Less Or Equal?(x=w1294, y=w1298) -> (x <= y?=w1296:bool)
                  n564 = Greater Or Equal?(x=w1294, y=5800.0) -> (x >= y?=w1295:bool)
                  n565 = property on="Stop Button" class="Bool (strict)"() -> ("Value"=w1291:bool)  [unwired: 2 in, 2 out]
                  n566 = Not(x=w1291) -> (.not. x?=w1290:bool)
                  n567 = Compound Arithmetic op=AND(w1296, w1295, w1290) -> (w1297:bool)
                  n568 = Add(x=w1298, y=w1301) -> (x+y=w1304:dbl)
                  n569 = Subtract(x=w1298, y=w1301) -> (x-y=w1305:dbl)
                  n570 = In Range and Coerce(upper limit=w1304, x=w1294, lower limit=w1305) -> (In Range?=w1289:bool)  [unwired: 1 out]
                  n571 = Compound Arithmetic op=OR(w1297, w1289) -> (w1299:bool)
                }
              }
              n572 = while {
                tunnel: w1227 -> [w1319]
                tunnel: w1250 -> [w1333]
                tunnel: [w1319] -> w1226
                tunnel: w1230 -> [w1320]
                stop <- w1318 stop-if-true
                n573 = control-ref of="Pannel User Message"() -> (w1321:refnum<vi>)
                n574 = property on="Stop Button" class="Bool (strict)"() -> ("Value"=w1317:bool)  [unwired: 2 in, 2 out]
                n575 = call <vilib>:"High Resolution Relative Seconds.vi"() -> ("relative seconds"=w1334:dbl)
                n576 = Subtract(x=w1334, y=w1333) -> (x-y=w1331:dbl)
                n577 = Subtract(x=4.0, y=w1331) -> (x-y=w1326:dbl)
                n578 = Less Or Equal To 0?(x=w1326) -> (x <= 0?=w1332:bool)
                n579 = Compound Arithmetic op=OR(w1332, w1317) -> (w1318:bool)
                n580 = Number To Fractional String(number=w1326, precision (6)=i16 2) -> (F-format string=w1328:string)  [unwired: 2 in]
                n581 = Concatenate Strings("7.5.6.Temperature controle test" ("Value"), "\r\n", "Time to wait: " ("Value"), w1328, "  Sec." ("string"), w1320) -> (w1323:string)
                n582 = property class="Str"(reference=w1321, "Value"=w1323) -> ()  [unwired: 1 in, 2 out]
              }
              n583 = call <vilib>:"High Resolution Relative Seconds.vi"() -> ("relative seconds"=w1254:dbl)
              n584 = Subtract(x=w1254, y=w1253) -> (x-y=w1252:dbl)
              n585 = Greater Or Equal?(x=w1252, y=180.0) -> (x >= y?=w1221:bool)
              n586 = Number To Fractional String(number=w1234, precision (6)=i16 2) -> (F-format string=w1239:string)  [unwired: 2 in]
              n587 = property on="Stop Button" class="Bool (strict)"() -> ("Value"=w1225:bool)  [unwired: 2 in, 2 out]
              n588 = Compound Arithmetic op=OR(w1244, w1245, w1221, w1225) -> (w1255:bool)
              n589 = First Call?() -> (First Call?: T/F=w1222:bool)
              n590 = Number To Fractional String(number=w1241, precision (6)=i16 2) -> (F-format string=w1237:string)  [unwired: 2 in]
              n591 = Concatenate Strings("\r\n", "Temp: " ("string"), w1239, "  Speed: " ("string"), w1237) -> (w1224:string)
              n592 = case shown="True" w1222 {
                tunnel: w1224 -> [w1260 _]
                tunnel: [w1260 ""] -> w1223
                frame False {
                }
                frame True {
                }
              }
            }
            n593 = case shown="False" w1152 {
              tunnel: [w1174 w1220] -> w1159
              tunnel: w1158 -> [w1173 _]
              tunnel: w1157 -> [w1172 _]
              tunnel: w1156 -> [w1171 w1220]
              tunnel: [w1168 w1219] -> w1155
              tunnel: w1151 -> [_ w1219]
              frame False {
                n594 = flat-sequence {
                  tunnel: w1171 -> [w1176]
                  tunnel: [w1176] -> w1170
                  tunnel: [w1175] -> w1169
                  frame #0 {
                    n595 = call <vilib>:"High Resolution Relative Seconds.vi"() -> ("relative seconds"=w1175:dbl)
                  }
                }
                n596 = while {
                  tunnel: w1170 -> [w1199]
                  tunnel: [w1198] -> w1174
                  tunnel: w1173 -> [w1197]
                  tunnel: w1172 -> [w1196]
                  tunnel: w1169 -> [w1191]
                  tunnel: [w1185] -> w1168
                  stop <- w1194 stop-if-true
                  w1181 = 120.0 ("y")
                  n597 = control-ref of="Motor Speed RPM"() -> (w1200:refnum<vi>)
                  n598 = control-ref of="Pannel User Message"() -> (w1190:refnum<vi>)
                  n599 = property class="DigNum (strict)"(reference=w1200, error in=w1199) -> (error out=w1198:errorcluster, "Value"=w1185:dbl)  [unwired: 1 out]
                  n600 = case shown="3, 4" w1196 {
                    tunnel: w1185 -> [w1202 w1208 w1214]
                    tunnel: [w1204 w1210 w1216] -> w1195
                    tunnel: w1197 -> [w1205 w1211 _]
                    frame 3, 4 {
                      n601 = Greater Or Equal?(x=w1202, y=5700.0) -> (x >= y?=w1203:bool)
                      n602 = Less Or Equal?(x=w1202, y=w1205) -> (x <= y?=w1206:bool)
                      n603 = And(x=w1203, y=w1206) -> (x .and. y?=w1204:bool)
                    }
                    frame 1, 2 {
                      n604 = Greater Or Equal?(x=w1208, y=w1211) -> (x >= y?=w1212:bool)
                      n605 = Less Or Equal?(x=w1208, y=15300.0) -> (x <= y?=w1209:bool)
                      n606 = And(x=w1212, y=w1209) -> (x .and. y?=w1210:bool)
                    }
                    frame Default {
                      n607 = Greater Or Equal?(x=w1214, y=5800.0) -> (x >= y?=w1218:bool)
                      n608 = Less Or Equal?(x=w1214, y=6200.0) -> (x <= y?=w1215:bool)
                      n609 = And(x=w1218, y=w1215) -> (x .and. y?=w1216:bool)
                    }
                  }
                  n610 = property on="Stop Button" class="Bool (strict)"() -> ("Value"=w1183:bool)  [unwired: 2 in, 2 out]
                  n611 = call <vilib>:"High Resolution Relative Seconds.vi"() -> ("relative seconds"=w1192:dbl)
                  n612 = Subtract(x=w1192, y=w1191) -> (x-y=w1180:dbl)
                  n613 = Number To Fractional String(number=w1185, precision (6)=i16 2) -> (F-format string=w1187:string)  [unwired: 2 in]
                  n614 = Subtract(x=w1181, y=w1180) -> (x-y=w1179:dbl)
                  n615 = Number To Fractional String(number=w1179, precision (6)=i16 2) -> (F-format string=w1177:string)  [unwired: 2 in]
                  n616 = Concatenate Strings("7.5.6.Temperature controle test\n" ("string"), "Motor speed [rpm]: " ("string"), w1187, "\nTimeout [sec]: " ("string"), w1177) -> (w1184:string)
                  n617 = property class="Str"(reference=w1190, "Value"=w1184) -> ()  [unwired: 1 in, 2 out]
                  n618 = Greater Or Equal?(x=w1180, y=w1181) -> (x >= y?=w1193:bool)
                  n619 = Compound Arithmetic op=OR(w1195, w1193, w1183) -> (w1194:bool)
                }
              }
              frame True {
              }
            }
          }
          frame Disabled {
            w1338 = TRUE ("Boolean")
          }
        }
        n620 = Number To Fractional String(number=w1128, precision (6)=i16 2) -> (F-format string=w1135:string)  [unwired: 2 in]
        n621 = Number To Fractional String(number=w1113, precision (6)=i16 2) -> (F-format string=w1144:string)  [unwired: 2 in]
        n622 = Increment(x=w1146) -> (x+1=w1131:i32)
        n623 = Multiply(x=2, y=w1114) -> (x*y=w1147:i32)
        n624 = Add(x=w1131, y=w1147) -> (x+y=w1133:i32)
        n625 = call "PassOrFail (SubVI).vi"("disabled index (col)"=w1130, "index (row)"=w1133, "error in (no error)"=w1116, "Boolean"=w1112, "Table in"=w1124) -> ("error out"=w1143:errorcluster)  [unwired: 6 in]
        n626 = property class="Tbl (strict)"(reference=w1139, error in=w1143) -> (reference out=w1142:refnum<vi>, error out=w1126:errorcluster, "Value"=w1145:string[][])
        n627 = Replace Array Subset(array=w1145, new element=w1144, index (row)=w1133, index (col)=5 ("disabled index (col)")) -> (w1127:string[][])
        n628 = property class="Tbl (strict)"(reference=w1124, error in=w1126, "Value"=w1127) -> (reference out=w1122:refnum<vi>, error out=w1125:errorcluster)
        n629 = Increment(x=w1133) -> (x+1=w1129:i32)
        n630 = call "PassOrFail (SubVI).vi"("disabled index (col)"=w1130, "index (row)"=w1129, "error in (no error)"=w1125, "Boolean"=w1111, "Table in"=w1124) -> ("error out"=w1123:errorcluster)  [unwired: 6 in]
        n631 = property class="Tbl (strict)"(reference=w1122, error in=w1123) -> (error out=w1120:errorcluster, "Value"=w1121:string[][])  [unwired: 1 out]
        n632 = Replace Array Subset(array=w1121, new element=w1135, index (row)=w1129, index (col)=5 ("disabled index (col)")) -> (w1134:string[][])
        n633 = property class="Tbl (strict)"(reference=w1142, error in=w1120, "Value"=w1134) -> (error out=w1138:errorcluster)  [unwired: 1 out]
      }
      n634 = property class="VISAName"(reference=w1068, error in=w1054) -> (error out=w1033:errorcluster, "Value"=w1071:refnum<visa-resource-name>)  [unwired: 1 out]
      n635 = property on="Property Node" class="Bool (strict)"(error in=w1033, "DisabledEnum"=w1034) -> (error out=w1035:errorcluster)  [unwired: 1 in, 1 out]
      n636 = property on="Property Node" class="Bool (strict)"(error in=w1035, "DisabledEnum"=w1034) -> (error out=w1031:errorcluster)  [unwired: 1 in, 1 out]
      n637 = VISA Write(VISA resource name=w1071, write buffer=w1070, error in (no error)=w1033) -> ()  [unwired: 3 out]
      n638 = property on="TempAlg" class="Bool (strict)"(error in=w1031, "Value"=FALSE ("TempAlg")) -> ()  [unwired: 1 in, 2 out]
      n639 = Build Array (concatenate)(w1041, w1040) -> (w1039:bool[])
      n640 = And Array Elements(Boolean array=w1039) -> (logical AND=→"TempControlind":bool)
    }
    frame "Burn in" {
      w1348 = TRUE ("rpm")
      w1350 = FALSE ("PrintTime")
      w1366 = T9."Enabled" ("Disabled")
      w1369 = T9."Disabled and Grayed Out" ("Disabled")
      (unwired) "EP=1r\nVC=15100\r\n" ("write buffer")
      (unwired) dbl[] [60.0, 60.0, 60.0]
      w1434 = 13.0 ("y")
      w1433 = 25.0 ("x")
      w1432 = 2 ("disabled index (col)")
      w1439 = 6 ("disabled index (col)")
      w1458 = 400.0 ("y")
      w1457 = 15100.0 ("x")
      w1364 = "7.5.7.Burn-in test in process" ("Value")
      w1343 = "7.5.7" ("Test Paragraph")
      # "k16+Venable"
      # "K15 + Venable + 90deg OFF"
      # "Venable"
      n641 = property on="Property Node" class="Bool (strict)"(error in=w1368, "DisabledEnum"=w1369) -> (error out=w1370:errorcluster)  [unwired: 1 in, 1 out]
      n642 = Byte Array To String(unsigned byte array=u8[] [75, 0, 4, 2, 0, 0, 2, 0] ("appended array")) -> ()  [unwired: 1 out]
      n643 = property on="Property Node" class="Bool (strict)"(error in=w1370, "DisabledEnum"=w1369) -> (error out=w1341:errorcluster)  [unwired: 1 in, 1 out]
      n644 = control-ref of="Pannel User Message"() -> (w1466:refnum<vi>)
      n645 = Concatenate Strings(w1364, "\nFull speed operation" ("string")) -> (w1363:string)
      n646 = property class="Str"(reference=w1466, error in=w1341, "Value"=w1364) -> (reference out=w1355:refnum<vi>, error out=w1397:errorcluster)
      n647 = property on="Property Node" class="DigNum (strict)"() -> ("Value"=w1377:dbl)  [unwired: 2 in, 2 out]
      n648 = control-ref of="VISA resource name out"() -> (w1471:refnum<vi>)
      n649 = property on="Property Node" class="Str"() -> ("Value"=w1347:string)  [unwired: 2 in, 2 out]
      n650 = control-ref of="Stop Button"() -> (w1356:refnum<vi>)
      n651 = control-ref of="Config_CANAT"() -> (w1384:refnum<vi>)
      n652 = control-ref of="Config_CANAT"() -> (w1392:refnum<vi>)
      n653 = control-ref of="Config_CANAT"() -> (w1399:refnum<vi>)
      n654 = control-ref of="UUT"() -> (w1385:refnum<vi>)
      n655 = control-ref of="Power transistor Heat sink Temp."() -> (w1435:refnum<vi>)
      n656 = control-ref of="UUT"() -> (w1391:refnum<vi>)
      n657 = control-ref of="UUT"() -> (w1400:refnum<vi>)
      n658 = control-ref of="Motor Speed RPM"() -> (w1464:refnum<vi>)
      n659 = control-ref of="Motor Speed RPM"() -> (w1349:refnum<vi>)
      n660 = Byte Array To String(unsigned byte array=u8[] [75, 0, 4, 2, 0, 0, 0, 0] ("appended array")) -> (string=w1474:string)
      n661 = Equal?(x=w1347, y="EBAY") -> (x = y?=w1345:bool)
      n662 = Add(x=w1457, y=w1458) -> (x+y=w1459:dbl)
      n663 = Add(x=w1433, y=w1434) -> (x+y=w1436:dbl)
      n664 = case shown="False" w1345 {
        tunnel: [28.0 ("x") 50.0 ("x")] -> w1450
        tunnel: [5.0 ("y") 7.0 ("y")] -> w1449
        frame False {
        }
        frame True {
        }
      }
      n665 = Add(x=w1450, y=w1449) -> (x+y=w1448:dbl)
      n666 = Subtract(x=w1457, y=w1458) -> (x-y=w1460:dbl)
      n667 = Subtract(x=w1433, y=w1434) -> (x-y=w1437:dbl)
      n668 = disable-structure shown="Enabled" {
        disable-tunnel: w1400 -> [w1592 _]
        disable-tunnel: w1399 -> [w1591 _]
        disable-tunnel: u16 0 ("Motor Speed RPM") -> [w1589 _]
        disable-tunnel: w1397 -> [w1588 w1593]
        disable-tunnel: [w1587 w1593] -> w1396
        frame Disabled {
          n669 = call "CANSendMotorSpeed.vi"("Remote"=FALSE, "error in (no error)"=w1588, "Motor Speed RPM"=w1589, "UUT"=w1592, "Cluster in"=w1591) -> ("error out"=w1587:errorcluster)  [unwired: 6 in]
        }
        frame Enabled {
        }
      }
      n670 = Byte Array To String(unsigned byte array=u8[] [75, 0, 4, 2, 0, 0, 2, 0] ("appended array")) -> (string=w1485:string)
      n671 = Subtract(x=w1450, y=w1449) -> (x-y=w1447:dbl)
      n672 = call "Reset old test Values (SubVI).vi"("error in"=w1396, "Atr in"=w1342, "Test Paragraph"=w1343) -> ("error out"=w1344:errorcluster)  [unwired: 8 in]
      n673 = call "Table_ScrollaBarMarvin.vi"("error in"=w1344, "Line to focus"=w1343, "reference in"=w1342) -> ("error out"=w1483:errorcluster)  [unwired: 2 out]
      n674 = property class="Tbl (strict)"(reference=w1342, error in=w1483) -> (reference out=w1413:refnum<vi>, error out=w1482:errorcluster, "Value"=w1481:string[][])
      n675 = Index Array(array=w1481, index (col)=0 ("disabled index (col)")) -> (element=w1480:string[])  [unwired: 1 in]
      n676 = call "Find_Number_LineMARVIN.vi"("Test Paragraph"=w1343, "error in"=w1482, "Row Headers[]"=w1480) -> ("error out"=w1478:errorcluster, "Line number"=w1452:i32)  [unwired: 2 in, 2 out]
      n677 = call "Table_ScrollaBarMarvin.vi"("error in"=w1478, "Line to focus"=w1343, "reference in"=w1413) -> ("error out"=w1477:errorcluster)  [unwired: 2 out]
      n678 = property class="VISAName"(reference=w1471, error in=w1477) -> (error out=w1486:errorcluster, "Value"=w1484:refnum<visa-resource-name>)  [unwired: 1 out]
      n679 = VISA Write(VISA resource name=w1484, write buffer=w1485, error in (no error)=w1486) -> (VISA resource name out=w1469:refnum<visa-resource-name>, error out=w1470:errorcluster)  [unwired: 1 out]
      n680 = call "Wait_Sec.vi"("Delay Time (sec)"=0.0, "error out"=w1470) -> ("error in"=w1380:errorcluster)  [unwired: 2 in]
      n681 = property class="DigNum (strict)"(reference=w1435, error in=w1380) -> (error out=w1379:errorcluster, "Value"=w1428:dbl)  [unwired: 1 out]
      n682 = In Range and Coerce(upper limit=w1436, x=w1428, lower limit=w1437) -> (In Range?=w1374:bool)  [unwired: 1 out]
      n683 = Number To Fractional String(number=w1428, precision (6)=i16 2) -> (F-format string=w1443:string)  [unwired: 2 in]
      n684 = call "Write panel message (SubVI).vi"("rpm"=w1349, "Stop"=w1356, "error in (no error)"=w1379, "Time to wait"=10.0 ("Delay Time (sec)"), "Strin"=w1364, "String in"=w1355) -> ("error out"=w1394:errorcluster)  [unwired: 5 in]
      n685 = call "CANSendMotorSpeed.vi"("Remote"=TRUE, "error in (no error)"=w1394, "Motor Speed RPM"=u16 15100, "UUT"=w1391, "Cluster in"=w1392) -> ("error out"=w1393:errorcluster)  [unwired: 6 in]
      n686 = call "Write panel message (SubVI).vi"(4:"rpm"=w1349, 5:"rpm"=w1348, "PrintTime"=w1350, "Stop"=w1356, "error in (no error)"=w1393, "Time to wait"=30.0 ("Delay Time (sec)"), "Strin"=w1363, "String in"=w1355) -> ("error out"=w1463:errorcluster)  [unwired: 3 in]
      n687 = call "Write panel message (SubVI).vi"(4:"rpm"=w1349, 5:"rpm"=w1348, "PrintTime"=w1350, "Stop"=w1356, "error in (no error)"=w1463, "Time to wait"=1.0, "Strin"="7.5.7.Burn-in test in process.\nDC current measure.", "String in"=w1355) -> ("error out"=w1357:errorcluster)  [unwired: 3 in]
      n688 = for {
        N: 10 -> [_]
        tunnel: w1469 -> [w1512]
        tunnel: [w1503] -> w1352 mode=indexing
        tunnel: w1357 -> [w1511]
        tunnel: [w1504] -> w1461
        stop <- w1501 stop-if-true
        # "Get Current by ADC (2)"
        n689 = flat-sequence {
          tunnel: w1507 -> [w1514]
          tunnel: [w1514] -> w1506
          tunnel: [w1513] -> w1505
          frame #0 {
            n690 = call <vilib>:"High Resolution Relative Seconds.vi"() -> ("relative seconds"=w1513:dbl)
          }
        }
        n691 = Byte Array To String(unsigned byte array=u8[] [75, 0, 4, 17, 0, 0, 0, 0] ("appended array")) -> (string=w1510:string)
        n692 = call "Time Delay6"("error in (no error)"=w1511) -> ("error out"=w1502:errorcluster)  [unwired: 10 in]
        n693 = VISA Write(VISA resource name=w1512, write buffer=w1510, error in (no error)=w1502) -> (VISA resource name out=w1508:refnum<visa-resource-name>, error out=w1507:errorcluster)  [unwired: 1 out]
        n694 = while {
          tunnel: w1508 -> [w1527]
          tunnel: w1506 -> [w1526]
          tunnel: [w1525] -> _
          tunnel: [w1524] -> w1504
          tunnel: w1505 -> [w1522]
          tunnel: [w1516] -> w1503
          stop <- w1518 stop-if-true
          n695 = call <vilib>:"High Resolution Relative Seconds.vi"() -> ("relative seconds"=w1523:dbl)
          n696 = Subtract(x=w1523, y=w1522) -> (x-y=w1521:dbl)
          n697 = Greater Or Equal?(x=w1521, y=10.0) -> (x >= y?=w1519:bool)
          n698 = property on="Stop Button" class="Bool (strict)"() -> ("Value"=w1515:bool)  [unwired: 2 in, 2 out]
          n699 = VISA Read(VISA resource name=w1527, byte count=u32 1, error in (no error)=w1526) -> (VISA resource name out=w1529:refnum<visa-resource-name>, read buffer=w1530:string, error out=w1528:errorcluster)  [unwired: 1 out]
          n700 = String To Byte Array(string=w1530) -> (unsigned byte array=w1533:u8[])
          n701 = Index Array(array=w1533, index=0) -> (element=w1531:u8)
          n702 = case shown="75" w1531 {
            tunnel: [w1538 w1542] -> w1524
            tunnel: w1529 -> [w1537 w1551]
            tunnel: w1528 -> [w1538 w1550]
            tunnel: [w1537 w1543] -> w1525
            tunnel: [u32 9999 w1540] -> w1516
            tunnel: [FALSE w1539] -> w1517
            frame 0, Default {
            }
            frame 75 {
              n703 = VISA Read(VISA resource name=w1551, byte count=u32 3, error in (no error)=w1550) -> (VISA resource name out=w1546:refnum<visa-resource-name>, read buffer=w1554:string, error out=w1545:errorcluster)  [unwired: 1 out]
              n704 = String To Byte Array(string=w1554) -> (unsigned byte array=w1544:u8[])
              n705 = Index Array(array=w1544, index #1=0 ("index")) -> (element #1=w1549:u8, element #2=w1547:u8)  [unwired: 2 in, 1 out]
              n706 = Equal?(x=u8 0, y=w1549) -> (x = y?=w1548:bool)
              n707 = case shown="True" w1548 {
                tunnel: [w1557 w1564] -> w1542
                tunnel: w1547 -> [_ w1571]
                tunnel: w1546 -> [w1558 w1570]
                tunnel: w1545 -> [w1557 w1569]
                tunnel: w1544 -> [_ w1568]
                tunnel: [w1558 w1566] -> w1543
                tunnel: [u32 9999 w1560] -> w1540
                tunnel: [FALSE w1559] -> w1539
                frame False {
                }
                frame True {
                  n708 = VISA Read(VISA resource name=w1570, byte count=w1571, error in (no error)=w1569) -> (VISA resource name out=w1566:refnum<visa-resource-name>, read buffer=w1565:string, error out=w1564:errorcluster)  [unwired: 1 out]
                  n709 = String To Byte Array(string=w1565) -> (unsigned byte array=w1567:u8[])
                  n710 = Insert Into Array(array=w1568, new element=w1567) -> (w1561:u8[])  [unwired: 1 in]
                  n711 = Index Array(array=w1561, index #1=0 ("index")) -> (element #3=w1562:u8)  [unwired: 2 in, 2 out]
                  n712 = case shown="15..19" w1562 {
                    tunnel: w1561 -> [_ w1585]
                    tunnel: [u32 9999 w1574] -> w1560
                    tunnel: [FALSE w1575] -> w1559
                    frame 0, Default {
                    }
                    frame 15..19 {
                      n713 = Index Array(array=w1585, index #1=3 ("index")) -> (element #1=w1584:u8, element #2=w1583:u8, element #3=w1582:u8, element #4=w1581:u8)  [unwired: 3 in]
                      n714 = Join Numbers(hi=w1581, lo=w1582) -> ((hi.lo)=w1579:u16)
                      n715 = Join Numbers(hi=w1583, lo=w1584) -> ((hi.lo)=w1580:u16)
                      n716 = Join Numbers(hi=w1579, lo=w1580) -> ((hi.lo)=w1577:u32)
                      n717 = Multiply(x=0.02003173828125, y=w1577) -> (x*y=w1574:dbl)
                      n718 = Greater Or Equal?(x=w1574, y=40.0) -> (x >= y?=w1575:bool)
                    }
                  }
                }
              }
            }
          }
          n719 = Compound Arithmetic op=OR(w1515, w1519, w1517) -> (w1518:bool)
        }
        n720 = property on="Stop Button" class="Bool (strict)"() -> ("Value"=w1501:bool)  [unwired: 2 in, 2 out]
      }
      n721 = for {
        tunnel: w1352 -> [_] mode=indexing
        shift-right: [w1491] -> w1351
        shift-left: w1352 -> [w1494]
        n722 = Search 1D Array(1D array=w1494, element=9999.0) -> (index of element=w1492:i32)  [unwired: 1 in]
        n723 = Greater Or Equal To 0?(x=w1492) -> (x >= 0?=w1493:bool)
        n724 = case shown="True" w1493 {
          tunnel: w1494 -> [w1496 w1499]
          tunnel: w1492 -> [_ w1498]
          tunnel: [w1496 w1497] -> w1491
          frame False {
          }
          frame True {
            n725 = Delete From Array(array=w1499, length=1, index=w1498) -> (deleted portion=w1497:dbl[])  [unwired: 1 out]
          }
        }
      }
      n726 = Add Array Elements(numeric array=w1351) -> (sum=w1360:dbl)
      n727 = Divide(x=w1360, y=10.0) -> (x/y=w1359:dbl)
      n728 = Subtract(x=w1359, y=w1377) -> (x-y=w1378:dbl)
      n729 = In Range and Coerce(upper limit=w1448, x=w1378, lower limit=w1447) -> (In Range?=w1373:bool)  [unwired: 1 out]
      n730 = call <vilib>:"Clear Errors.vi"("error in (no error)"=w1461) -> ("error out"=w1388:errorcluster)  [unwired: 5 in, 1 out]
      n731 = property class="DigNum (strict)"(reference=w1464, error in=w1388) -> (error out=w1381:errorcluster, "Value"=w1423:dbl)  [unwired: 1 out]
      n732 = In Range and Coerce(upper limit=w1459, x=w1423, lower limit=w1460) -> (In Range?=w1375:bool)  [unwired: 1 out]
      n733 = Number To Fractional String(number=w1423, precision (6)=i16 2) -> (F-format string=w1444:string)  [unwired: 2 in]
      n734 = property class="Tbl (strict)"(reference=w1413, error in=w1381) -> (reference out=w1451:refnum<vi>, error out=w1408:errorcluster, "Value"=w1456:string[][])
      n735 = Number To Fractional String(number=w1378, precision (6)=i16 2) -> (F-format string=w1455:string)  [unwired: 2 in]
      n736 = Add(x=w1428, y=25.0) -> (x+y=w1422:dbl)
      n737 = Number To Fractional String(number=w1422, precision (6)=i16 2) -> (F-format string=w1426:string)  [unwired: 2 in]
      n738 = Concatenate Strings("< " ("string"), w1426) -> (w1425:string)
      n739 = Increment(x=w1452) -> (x+1=w1440:i32)
      n740 = Replace Array Subset(array=w1456, new element=w1455, index (row)=w1440, index (col)=5 ("disabled index (col)")) -> (w1416:string[][])
      n741 = property class="Tbl (strict)"(reference=w1413, error in=w1408, "Value"=w1416) -> (reference out=w1415:refnum<vi>, error out=w1407:errorcluster)
      n742 = call "PassOrFail (SubVI).vi"("disabled index (col)"=w1439, "index (row)"=w1440, "error in (no error)"=w1407, "Boolean"=w1373, "Table in"=w1451) -> ("error out"=w1406:errorcluster)  [unwired: 6 in]
      n743 = property class="Tbl (strict)"(reference=w1415, error in=w1406) -> (reference out=w1411:refnum<vi>, error out=w1405:errorcluster, "Value"=w1414:string[][])
      n744 = Increment(x=w1440) -> (x+1=w1438:i32)
      n745 = Replace Array Subset(array=w1414, new element=w1444, index (row)=w1438, index (col)=5 ("disabled index (col)")) -> (w1412:string[][])
      n746 = property class="Tbl (strict)"(reference=w1411, error in=w1405, "Value"=w1412) -> (reference out=w1410:refnum<vi>, error out=w1404:errorcluster)
      n747 = call "PassOrFail (SubVI).vi"("disabled index (col)"=w1439, "index (row)"=w1438, "error in (no error)"=w1404, "Boolean"=w1375, "Table in"=w1413) -> ("error out"=w1403:errorcluster)  [unwired: 6 in]
      n748 = property class="Tbl (strict)"(reference=w1410, error in=w1403) -> (error out=w1402:errorcluster, "Value"=w1409:string[][])  [unwired: 1 out]
      n749 = Increment(x=w1438) -> (x+1=w1419:i32)
      n750 = Increment(x=w1419) -> (x+1=w1431:i32)
      n751 = Increment(x=w1431) -> (x+1=w1430:i32)
      n752 = Increment(x=w1430) -> (x+1=w1418:i32)
      n753 = Replace Array Subset(array=w1409, new element #1=w1443, index (row) #1=w1419, index (col) #1=5 ("disabled index (col)"), new element #2=w1425, index (row) #2=w1431, index (col) #2=w1432, new element #3=w1425, index (row) #3=w1430, index (col) #3=w1432, new element #4=w1425, index (row) #4=w1418, index (col) #4=w1432) -> (w1441:string[][])
      n754 = property class="Tbl (strict)"(reference=w1413, error in=w1402, "Value"=w1441) -> (error out=w1401:errorcluster)  [unwired: 1 out]
      n755 = call "PassOrFail (SubVI).vi"("disabled index (col)"=w1439, "index (row)"=w1419, "error in (no error)"=w1401, "Boolean"=w1374, "Table in"=w1413) -> ("error out"=w1340:errorcluster)  [unwired: 6 in]
      n756 = property on="Stop Burn-in" class="Bool"(error in=w1340, "Visible"=TRUE) -> (error out=w1339:errorcluster)  [unwired: 1 in, 1 out]
      n757 = for {
        tunnel: w1339 -> [w1618]
        tunnel: dbl[] [600.0, 600.0, 600.0] -> [w1615] mode=indexing
        tunnel: w1422 -> [w1612]
        tunnel: w1419 -> [w1609]
        tunnel: w1342 -> [w1603]
        tunnel: [w1595] -> w1383
        tunnel: [w1594] -> w1376 mode=indexing
        i -> [w1608]
        n758 = control-ref of="Power transistor Heat sink Temp."() -> (w1614:refnum<vi>)
        n759 = Increment(x=w1608) -> (x+1=w1607:i32)
        n760 = Add(x=w1609, y=w1607) -> (x+y=w1601:i32)
        n761 = flat-sequence {
          tunnel: [w1642] -> _
          tunnel: [w1642] -> w1617
          tunnel: [w1643] -> w1616
          tunnel: w1618 -> [w1642]
          frame #0 {
            n762 = call <vilib>:"High Resolution Relative Seconds.vi"() -> ("relative seconds"=w1643:dbl)
          }
        }
        n763 = while {
          tunnel: w1617 -> [w1637]
          tunnel: w1616 -> [w1640]
          tunnel: w1615 -> [w1631]
          tunnel: [w1628] -> w1613
          stop <- w1627 stop-if-true
          w1625 = i16 2 ("precision (6)")
          n764 = control-ref of="Pannel User Message"() -> (w1636:refnum<vi>)
          n765 = call <vilib>:"High Resolution Relative Seconds.vi"() -> ("relative seconds"=w1641:dbl)
          n766 = property on="Stop Button" class="Bool (strict)"() -> ("Value"=w1626:bool)  [unwired: 2 in, 2 out]
          n767 = Subtract(x=w1641, y=w1640) -> (x-y=w1630:dbl)
          n768 = Greater Or Equal?(x=w1630, y=w1631) -> (x >= y?=w1639:bool)
          n769 = Compound Arithmetic op=OR(w1626, "Stop Burn-in", w1639) -> (w1627:bool)
          n770 = Subtract(x=w1631, y=w1630) -> (x-y=w1632:dbl)
          n771 = Number To Fractional String(number=w1632, precision (6)=i16 2) -> (F-format string=w1633:string)  [unwired: 2 in]
          n772 = property on="Power transistor Heat sink Temp." class="DigNum (strict)"() -> ("Value"=w1624:dbl)  [unwired: 2 in, 2 out]
          n773 = Number To Fractional String(number=w1624, precision (6)=w1625) -> (F-format string=w1621:string)  [unwired: 2 in]
          n774 = property on="Motor Speed RPM" class="DigNum (strict)"() -> ("Value"=w1623:dbl)  [unwired: 2 in, 2 out]
          n775 = Number To Fractional String(number=w1623, precision (6)=w1625) -> (F-format string=w1619:string)  [unwired: 2 in]
          n776 = Concatenate Strings("Remained Time: " ("string"), w1633, "\nPCB Temp. [Deg]: " ("string"), w1621, "\nMotor speed [rpm]: " ("string"), w1619) -> (w1629:string)
          n777 = property class="Str"(reference=w1636, error in=w1637, "Value"=w1629) -> (error out=w1628:errorcluster)  [unwired: 1 out]
        }
        n778 = property class="DigNum (strict)"(reference=w1614, error in=w1613) -> (error out=w1604:errorcluster, "Value"=w1605:dbl)  [unwired: 1 out]
        n779 = Less Or Equal?(x=w1605, y=w1612) -> (x <= y?=w1594:bool)
        n780 = property class="Tbl (strict)"(reference=w1603, error in=w1604) -> (reference out=w1598:refnum<vi>, error out=w1597:errorcluster, "Value"=w1600:string[][])
        n781 = Number To Fractional String(number=w1605, precision (6)=i16 2) -> (F-format string=w1606:string)  [unwired: 2 in]
        n782 = Replace Array Subset(array=w1600, new element=w1606, index (row)=w1601, index (col)=5 ("disabled index (col)")) -> (w1599:string[][])
        n783 = property class="Tbl (strict)"(reference=w1598, error in=w1597, "Value"=w1599) -> (error out=w1596:errorcluster)  [unwired: 1 out]
        n784 = call "PassOrFail (SubVI).vi"("disabled index (col)"=6, "index (row)"=w1601, "error in (no error)"=w1596, "Boolean"=w1594, "Table in"=w1598) -> ("error out"=w1595:errorcluster)  [unwired: 6 in]
      }
      n785 = call "CANSendMotorSpeed.vi"("Remote"=FALSE, "error in (no error)"=w1383, "Motor Speed RPM"=u16 0, "UUT"=w1385, "Cluster in"=w1384) -> ("error out"=w1382:errorcluster)  [unwired: 6 in]
      n786 = property on="Stop Burn-in" class="Bool"(error in=w1382, "Visible"=FALSE) -> (error out=w1365:errorcluster)  [unwired: 1 in, 1 out]
      n787 = property on="Property Node" class="Bool (strict)"(error in=w1365, "DisabledEnum"=w1366) -> (error out=w1367:errorcluster)  [unwired: 1 in, 1 out]
      n788 = property on="Property Node" class="Bool (strict)"(error in=w1367, "DisabledEnum"=w1366) -> ()  [unwired: 1 in, 2 out]
      n789 = property class="VISAName"(reference=w1471, error in=w1365) -> (error out=w1473:errorcluster, "Value"=w1475:refnum<visa-resource-name>)  [unwired: 1 out]
      n790 = VISA Write(VISA resource name=w1475, write buffer=w1474, error in (no error)=w1473) -> ()  [unwired: 3 out]
      n791 = Build Array (concatenate)(w1376, w1375, w1374, w1373) -> (w1372:bool[])
      n792 = And Array Elements(Boolean array=w1372) -> (logical AND=→"Burninind":bool)
    }
    frame "Visual Inspec" {
      w1647 = T9."Enabled" ("Disabled")
      w1650 = T9."Disabled and Grayed Out" ("Disabled")
      n793 = property on="Property Node" class="Bool (strict)"(error in=w1649, "DisabledEnum"=w1650) -> (error out=w1651:errorcluster)  [unwired: 1 in, 1 out]
      n794 = property on="Property Node" class="Bool (strict)"(error in=w1651, "DisabledEnum"=w1650) -> (error out=w1648:errorcluster)  [unwired: 1 in, 1 out]
      n795 = call "VisualInspection.vi"("error in (no error)"=w1648, "TableRef"=w1653) -> ("error out"=w1645:errorcluster, "VisualInspectionResult"=w1652:bool)  [unwired: 8 in]
      "VisualInspectionResult" <- w1652
      n796 = property on="Property Node" class="Bool (strict)"() -> ("Value"=w1644:bool)  [unwired: 2 in, 2 out]
      n797 = property on="Property Node" class="Bool (strict)"(error in=w1645, "DisabledEnum"=w1647) -> (error out=w1646:errorcluster)  [unwired: 1 in, 1 out]
      n798 = property on="Property Node" class="Bool (strict)"(error in=w1646, "DisabledEnum"=w1647) -> ()  [unwired: 1 in, 2 out]
      n799 = case shown="True" w1644 {
        tunnel: w1652 -> [_ w1654]
        frame False {
        }
        frame True {
          n800 = property on="Property Node" class="Bool (strict)"("Val(Sgnl)"=w1654) -> ()  [unwired: 2 in, 2 out]
        }
      }
    }
    frame "Temp Sens Cal" {
      w1686 = T9."Enabled" ("Disabled")
      w1690 = T9."Disabled and Grayed Out" ("Disabled")
      w1665 = "7.5.5.Temperature sensor calibration test in process..." ("Value")
      w1670 = FALSE ("Clear Log")
      w1657 = "7.5.5" ("Test Paragraph")
      # "K15 OFF + Venable"
      # "K15 OFF + Venable"
      n801 = property on="Property Node" class="Bool (strict)"(error in=w1689, "DisabledEnum"=w1690) -> (error out=w1691:errorcluster)  [unwired: 1 in, 1 out]
      n802 = property on="Property Node" class="Bool (strict)"(error in=w1691, "DisabledEnum"=w1690) -> (error out=w1688:errorcluster)  [unwired: 1 in, 1 out]
      n803 = VISA Flush I/O Buffer(VISA resource name=w1694, error in (no error)=w1688) -> (VISA resource name out=w1673:refnum<visa-resource-name>, error out=w1693:errorcluster)  [unwired: 1 in]
      n804 = control-ref of="VISA resource name out"() -> (w1681:refnum<vi>)
      n805 = control-ref of="Config_CANAT"() -> (w1660:refnum<vi>)
      n806 = control-ref of="UUT"() -> (w1661:refnum<vi>)
      n807 = control-ref of="Pannel User Message"() -> (w1696:refnum<vi>)
      n808 = Byte Array To String(unsigned byte array=u8[] [75, 0, 4, 2, 0, 0, 0, 0] ("appended array")) -> (string=w1675:string)
      n809 = Concatenate Strings("EP=1\r\nAO" ("string"), "[", "1" ("string"), "]=0", "\r\n" ("write buffer")) -> (w1700:string)
      n810 = Byte Array To String(unsigned byte array=u8[] [75, 0, 4, 2, 0, 0, 16, 0] ("appended array")) -> (string=w1682:string)
      n811 = property class="Str"(reference=w1696, error in=w1693, "Value"=w1665) -> (error out=w1695:errorcluster)  [unwired: 1 out]
      n812 = call "Reset old test Values (SubVI).vi"("error in"=w1695, "Atr in"=w1656, "Test Paragraph"=w1657) -> ("error out"=w1658:errorcluster)  [unwired: 8 in]
      n813 = call "Table_ScrollaBarMarvin.vi"("error in"=w1658, "Line to focus"=w1657, "reference in"=w1656) -> ("error out"=w1707:errorcluster)  [unwired: 2 out]
      n814 = property class="Tbl (strict)"(reference=w1656, error in=w1707) -> (error out=w1709:errorcluster, "Value"=w1710:string[][])  [unwired: 1 out]
      n815 = Index Array(array=w1710, index (col)=0 ("disabled index (col)")) -> (element=w1711:string[])  [unwired: 1 in]
      n816 = call "Find_Number_LineMARVIN.vi"("Test Paragraph"=w1657, "error in"=w1709, "Row Headers[]"=w1711) -> ("error out"=w1706:errorcluster, "Line number"=w1704:i32)  [unwired: 2 in, 2 out]
      n817 = property on="Property Node" class="Bool (strict)"(error in=w1706) -> (error out=w1699:errorcluster, "Value"=w1705:bool)  [unwired: 1 in, 1 out]
      n818 = call "CANSendMotorSpeed.vi"("Remote"=TRUE, "error in (no error)"=w1699, "Motor Speed RPM"=u16 0, "UUT"=w1661, "Cluster in"=w1660) -> ("error out"=w1664:errorcluster)  [unwired: 6 in]
      n819 = call "Time Delay10"("error in (no error)"=w1664) -> ("error out"=w1659:errorcluster)  [unwired: 10 in]
      n820 = call "SerialMarvinMod.vi"("error in (no error)"=w1659, "Clear Log"=w1670, "write buffer"=w1700, "VISA resource name"=w1673) -> ("error out"=w1679:errorcluster)  [unwired: 6 in, 1 out]
      n821 = property class="VISAName"(reference=w1681, error in=w1679) -> (error out=w1683:errorcluster, "Value"=w1684:refnum<visa-resource-name>)  [unwired: 1 out]
      n822 = VISA Write(VISA resource name=w1684, write buffer=w1682, error in (no error)=w1683) -> (VISA resource name out=w1674:refnum<visa-resource-name>, error out=w1677:errorcluster)  [unwired: 1 out]
      n823 = call "Time Delay9"("error in (no error)"=w1677) -> ("error out"=w1676:errorcluster)  [unwired: 10 in]
      n824 = VISA Write(VISA resource name=w1674, write buffer=w1675, error in (no error)=w1676) -> (error out=w1671:errorcluster)  [unwired: 2 out]
      n825 = call "SerialMarvinMod.vi"("error in (no error)"=w1671, "Clear Log"=w1670, "write buffer"="AO[1]\r\n", "VISA resource name"=w1673) -> ("error out"=w1655:errorcluster, "read buffer"=w1669:string)  [unwired: 6 in]
      n826 = Equal?(x=w1669, y="") -> (x = y?=w1666:bool)
      n827 = And(x=w1705, y=w1666) -> (x .and. y?=w1667:bool)
      n828 = case shown="True" w1667 {
        selector: w1667 -> [w1713 _]
        tunnel: w1655 -> [w1718 _]
        tunnel: w1656 -> [w1717 w1754]
        tunnel: w1704 -> [w1716 w1753]
        tunnel: w1673 -> [_ w1757]
        tunnel: [w1713 w1745] -> w1692
        tunnel: [w1712 w1724] -> w1685
        tunnel: w1665 -> [_ w1742]
        tunnel: w1655 -> [_ w1741]
        frame False {
          n829 = flat-sequence {
            tunnel: w1718 -> [w1719]
            tunnel: [w1719] -> w1712
            frame #0 {
              n830 = One Button Dialog(message="Please establish RS connection.") -> ()  [unwired: 1 in, 1 out]
            }
          }
          n831 = Increment(x=w1716) -> (x+1=w1715:i32)
          n832 = call "PassOrFail (SubVI).vi"("disabled index (col)"=6, "index (row)"=w1715, "error in (no error)"=w1712, "Boolean"=w1713, "Table in"=w1717) -> ()  [unwired: 6 in, 1 out]
        }
        frame True {
          (unwired) dbl[] [0.68545] ("Val 2")
          (unwired) dbl[] [0.69103] ("Val 2")
          (unwired) u32[] [2048]
          # "Max"
          n833 = for {
            tunnel: u32[] [64, 512, 2048, 8192] -> [w1830] mode=indexing
            tunnel: w1757 -> [w1859]
            tunnel: dbl[] [0.59774, 0.65238, 0.68545, 0.71584] ("Val 2") -> [w1819] mode=indexing
            tunnel: [w1816] -> w1792 mode=indexing
            tunnel: [w1858] -> w1786
            tunnel: [w1834] -> w1737
            tunnel: [w1816] -> w1751 mode=indexing
            tunnel: [w1857] -> w1748 mode=indexing
            tunnel: dbl[] [0.60155, 0.65733, 0.69103, 0.72203] ("Val 2") -> [w1855] mode=indexing
            tunnel: [w1856] -> w1744 mode=indexing
            tunnel: [w1853] -> w1743 mode=indexing
            tunnel: w1742 -> [w1852]
            tunnel: w1741 -> [w1825]
            n834 = control-ref of="VISA resource name out"() -> (w1844:refnum<vi>)
            n835 = control-ref of="Stop Button"() -> (w1850:refnum<vi>)
            n836 = control-ref of="Motor Speed RPM"() -> (w1851:refnum<vi>)
            n837 = control-ref of="Pannel User Message"() -> (w1849:refnum<vi>)
            n838 = To Unsigned Long Integer(number=w1830) -> (unsigned 32bit integer=w1841:u32)
            n839 = Split Number(x=w1841) -> (hi(x)=w1836:u16, lo(x)=w1835:u16)
            n840 = Split Number(x=w1835) -> (hi(x)=w1837:u8, lo(x)=w1838:u8)
            n841 = Split Number(x=w1836) -> (hi(x)=w1839:u8, lo(x)=w1840:u8)
            n842 = Build Array(u8 75, u8 0 ("element"), u8 4 ("Length"), u8 2, w1838, w1837, w1840, w1839) -> (w1842:u8[])
            n843 = Byte Array To String(unsigned byte array=w1842) -> (string=w1843:string)
            n844 = call "Write panel message (SubVI).vi"("rpm"=w1851, "PrintTime"=FALSE, "Stop"=w1850, "error in (no error)"=w1825, "Time to wait"=0.1, "Strin"="7.5.5.Temperature sensor calibration test in process...", "String in"=w1849) -> ("error out"=w1848:errorcluster)  [unwired: 4 in]
            n845 = property class="VISAName"(reference=w1844, error in=w1848) -> (error out=w1845:errorcluster, "Value"=w1834:refnum<visa-resource-name>)  [unwired: 1 out]
            n846 = VISA Flush I/O Buffer(VISA resource name=w1834, error in (no error)=w1845) -> (VISA resource name out=w1847:refnum<visa-resource-name>, error out=w1846:errorcluster)  [unwired: 1 in]
            n847 = VISA Write(VISA resource name=w1847, write buffer=w1843, error in (no error)=w1846) -> (error out=w1824:errorcluster)  [unwired: 2 out]
            n848 = call "Time Delay7"("error in (no error)"=w1824) -> ("error out"=w1823:errorcluster)  [unwired: 10 in]
            n849 = while {
              tunnel: w1859 -> [w1893]
              tunnel: [w1863] -> _
              tunnel: [w1891] -> w1857
              tunnel: [w1861] -> w1822
              tunnel: w1819 -> [w1862]
              tunnel: [w1878] -> w1856
              tunnel: w1855 -> [w1879]
              tunnel: [w1892] -> w1858
              shift-right: [w1871] -> w1853
              shift-left: 0.0 -> [w1872]
              tunnel: w1852 -> [w1869]
              tunnel: w1823 -> [w1865]
              tunnel: [w1864] -> w1821 mode=indexing
              i -> [w1876]
              stop <- w1877 stop-if-true
              n850 = control-ref of="Stop Button"() -> (w1867:refnum<vi>)
              n851 = control-ref of="Motor Speed RPM"() -> (w1866:refnum<vi>)
              n852 = control-ref of="Pannel User Message"() -> (w1868:refnum<vi>)
              n853 = Equal?(x=w1876, y=10) -> (x = y?=w1874:bool)
              n854 = property on="Stop Button" class="Bool (strict)"() -> ("Value"=w1873:bool)  [unwired: 2 in, 2 out]
              n855 = Compound Arithmetic op=OR(w1873, w1874) -> (w1877:bool)
              n856 = Concatenate Strings("TA" ("string"), "[", "Index", "]", "\r\n" ("write buffer")) -> (w1885:string)
              n857 = call "Write panel message (SubVI).vi"("rpm"=w1866, "PrintTime"=FALSE, "Stop"=w1867, "error in (no error)"=w1865, "Time to wait"=0.5 ("Delay Time (sec)"), "Strin"=w1869, "String in"=w1868) -> ("error out"=w1883:errorcluster)  [unwired: 4 in]
              n858 = call "SerialMarvinMod.vi"("error in (no error)"=w1883, "Clear Log"=FALSE, "write buffer"=w1885, "VISA resource name"=w1893) -> ("error out"=w1892:errorcluster, "read buffer"=w1891:string)  [unwired: 6 in]
              n859 = Fract/Exp String To Number(string=w1891) -> (number=w1864:dbl)  [unwired: 3 in, 1 out]
              n860 = Subtract(x=w1864, y=w1862) -> (x-y=w1863:dbl)
              n861 = Multiply(x=w1862, y=0.015) -> (x*y=w1880:dbl)
              n862 = Subtract(x=w1862, y=w1880) -> (x-y=w1878:dbl)
              n863 = In Range and Coerce(upper limit=w1879, x=w1864, lower limit=w1878) -> (In Range?=w1860:bool)  [unwired: 1 out]
              n864 = case shown="True" w1860 {
                tunnel: w1864 -> [w1895 w1898]
                tunnel: [w1894 w1897] -> w1861
                tunnel: w1872 -> [w1896 w1899]
                tunnel: [w1894 w1897] -> w1871
                frame False {
                  n865 = Max & Min(x=w1896, y=w1895) -> (max(x,y)=w1894:dbl)  [unwired: 1 out]
                }
                frame True {
                  n866 = Max & Min(x=w1899, y=w1898) -> (max(x,y)=w1897:dbl)  [unwired: 1 out]
                }
              }
            }
            n867 = Add Array Elements(numeric array=w1821) -> (sum=w1820:dbl)
            n868 = Divide(x=w1820, y=11.0 ("x")) -> (x/y=w1818:dbl)
            n869 = Subtract(x=w1822, y=w1819) -> ()  [unwired: 1 out]
            n870 = Subtract(x=w1818, y=w1819) -> (x-y=w1816:dbl)
          }
          "Array 2" <- w1751
          "Array 3" <- w1748
          "Array 4" <- w1744
          "Array 5" <- w1743
          n871 = control-ref of="Stop Button"() -> (w1736:refnum<vi>)
          n872 = control-ref of="Motor Speed RPM"() -> (w1734:refnum<vi>)
          n873 = control-ref of="Pannel User Message"() -> (w1735:refnum<vi>)
          n874 = To Unsigned Long Integer(number=u32 0) -> (unsigned 32bit integer=w1774:u32)
          n875 = Split Number(x=w1774) -> (hi(x)=w1780:u16, lo(x)=w1781:u16)
          n876 = Split Number(x=w1781) -> (hi(x)=w1779:u8, lo(x)=w1778:u8)
          n877 = Add Array Elements(numeric array=w1792) -> (sum=w1791:dbl)
          n878 = Divide(x=w1791, y=4.0) -> (x/y=w1750:dbl)
          n879 = In Range and Coerce(upper limit=0.1, x=w1750, lower limit=-0.1) -> (In Range?=w1746:bool)  [unwired: 1 out]
          n880 = And(x=w1746, y=w1746) -> (x .and. y?=w1745:bool)
          n881 = Number To Fractional String(number=w1750, precision (6)=i16 7) -> (F-format string=w1749:string)  [unwired: 2 in]
          n882 = Concatenate Strings("EP=1\r\nAO" ("string"), "[", "1" ("string"), "]=", w1749, "\r\n" ("write buffer")) -> (w1760:string)
          n883 = Increment(x=w1753) -> (x+1=w1765:i32)
          n884 = call "PassOrFail (SubVI).vi"("disabled index (col)"=6, "index (row)"=w1765, "error in (no error)"=w1786, "Boolean"=w1746, "Table in"=w1754) -> ("error out"=w1767:errorcluster)  [unwired: 6 in]
          n885 = property class="Tbl (strict)"(reference=w1754, error in=w1767) -> (reference out=w1771:refnum<vi>, error out=w1770:errorcluster, "Value"=w1768:string[][])
          n886 = Number To Fractional String(number=w1750, precision (6)=i16 4) -> (F-format string=w1755:string)  [unwired: 2 in]
          n887 = Replace Array Subset(array=w1768, new element=w1755, index (row)=w1765, index (col)=5 ("disabled index (col)")) -> (w1769:string[][])
          n888 = property class="Tbl (strict)"(reference=w1771, error in=w1770, "Value"=w1769) -> (error out=w1727:errorcluster)  [unwired: 1 out]
          n889 = case shown="True" w1746 {
            tunnel: w1760 -> [_ w1804]
            tunnel: w1727 -> [w1794 w1803]
            tunnel: w1757 -> [w1793 w1798]
            tunnel: ["0" ("read buffer") w1796] -> w1756
            tunnel: [w1794 w1800] -> w1726
            frame False {
              n890 = VISA Flush I/O Buffer(VISA resource name=w1793, error in (no error)=w1794) -> ()  [unwired: 1 in, 2 out]
            }
            frame True {
              n891 = call "SerialMarvinMod.vi"("error in (no error)"=w1803, "Clear Log"=FALSE, "write buffer"=w1804, "VISA resource name"=w1798) -> ("error out"=w1802:errorcluster)  [unwired: 6 in, 1 out]
              n892 = disable-structure shown="Enabled" {
                disable-tunnel: w1802 -> [w1812 w1815]
                disable-tunnel: [w1809 w1813] -> w1800
                disable-tunnel: "AO[1]\r\n" ("write buffer") -> [w1808 _]
                disable-tunnel: w1798 -> [w1807 w1814]
                disable-tunnel: FALSE ("Clear Log") -> [w1806 _]
                disable-tunnel: [w1805 _] -> w1796
                frame Disabled {
                  n893 = call "Time Delay8"("error in (no error)"=w1812) -> ("error out"=w1811:errorcluster)  [unwired: 10 in]
                  n894 = call "SerialMarvinMod.vi"("error in (no error)"=w1811, "Clear Log"=w1806, "write buffer"=w1808, "VISA resource name"=w1807) -> ("error out"=w1810:errorcluster)  [unwired: 6 in, 1 out]
                  n895 = call "SerialMarvinMod.vi"("error in (no error)"=w1810, "Clear Log"=w1806, "write buffer"=w1808, "VISA resource name"=w1807) -> ("error out"=w1809:errorcluster, "read buffer"=w1805:string)  [unwired: 6 in]
                }
                frame Enabled {
                  n896 = VISA Flush I/O Buffer(VISA resource name=w1814, error in (no error)=w1815) -> (error out=w1813:errorcluster)  [unwired: 1 in, 1 out]
                }
              }
            }
          }
          n897 = Equal?(x=w1749, y=w1756) -> ()  [unwired: 1 out]
          n898 = Split Number(x=w1780) -> (hi(x)=w1777:u8, lo(x)=w1776:u8)
          n899 = Build Array(u8 75, u8 0 ("element"), u8 4 ("Length"), u8 2, w1778, w1779, w1776, w1777) -> (w1772:u8[])
          n900 = Byte Array To String(unsigned byte array=w1772) -> (string=w1785:string)
          n901 = Byte Array To String(unsigned byte array=u8[] [75, 0, 4, 2, 0, 0, 16, 0] ("appended array")) -> (string=w1740:string)
          n902 = VISA Write(VISA resource name=w1737, write buffer=w1740, error in (no error)=w1726) -> (error out=w1738:errorcluster)  [unwired: 2 out]
          n903 = call <vilib>:"Clear Errors.vi"("error in (no error)"=w1738) -> ("error out"=w1731:errorcluster)  [unwired: 5 in, 1 out]
          n904 = call "Write panel message (SubVI).vi"(4:"rpm"=w1734, 5:"rpm"=FALSE ("rpm"), "PrintTime"=TRUE, "Stop"=w1736, "error in (no error)"=w1731, "Time to wait"=15.0, "Strin"="7.5.5.Temperature sensor calibration test in process...", "String in"=w1735) -> ("error out"=w1728:errorcluster)  [unwired: 3 in]
          n905 = VISA Write(VISA resource name=w1737, write buffer=w1785, error in (no error)=w1728) -> (error out=w1725:errorcluster)  [unwired: 2 out]
          n906 = call <vilib>:"Clear Errors.vi"("error in (no error)"=w1725) -> ("error out"=w1724:errorcluster)  [unwired: 5 in, 1 out]
          n907 = call "PassOrFail (SubVI).vi"("disabled index (col)"=6, "index (row)"=w1753, "error in (no error)"=w1724, "Boolean"=w1746, "Table in"=w1754) -> ()  [unwired: 6 in, 1 out]
        }
      }
      "TempSensCalind" <- w1692
      n908 = property on="Property Node" class="Bool (strict)"(error in=w1685, "DisabledEnum"=w1686) -> (error out=w1687:errorcluster)  [unwired: 1 in, 1 out]
      n909 = property on="Property Node" class="Bool (strict)"(error in=w1687, "DisabledEnum"=w1686) -> ()  [unwired: 1 in, 2 out]
    }
    frame "Auxiliary" {
      w1907 = T9."Enabled" ("Disabled")
      w1911 = T9."Disabled and Grayed Out" ("Disabled")
      w1904 = "8.Auxiliary test" ("Value")
      w1902 = "8" ("Test Paragraph")
      # "K20 OFF"
      # "K20 ON"
      # "OFF"
      n910 = property on="Property Node" class="Bool (strict)"(error in=w1910, "DisabledEnum"=w1911) -> (error out=w1912:errorcluster)  [unwired: 1 in, 1 out]
      n911 = property on="Property Node" class="Bool (strict)"(error in=w1912, "DisabledEnum"=w1911) -> (error out=w1909:errorcluster)  [unwired: 1 in, 1 out]
      n912 = control-ref of="Pannel User Message"() -> (w1926:refnum<vi>)
      n913 = property class="Str"(reference=w1926, error in=w1909, "Value"=w1904) -> (reference out=w1905:refnum<vi>, error out=w1925:errorcluster)
      n914 = control-ref of="VISA resource name out"() -> (w1929:refnum<vi>)
      n915 = Build Array(u8[] [75, 0, 4, 2, 0, 0, 8, 0] ("appended array"), u8[] [75, 0, 4, 2, 0, 0, 0, 0] ("appended array")) -> (w1921:u8[][])
      n916 = Byte Array To String(unsigned byte array=u8[] [75, 0, 4, 2, 0, 0, 0, 0] ("appended array")) -> (string=w1931:string)
      n917 = call "Reset old test Values (SubVI).vi"("error in"=w1925, "Atr in"=w1901, "Test Paragraph"=w1902) -> ("error out"=w1903:errorcluster)  [unwired: 8 in]
      n918 = call "Table_ScrollaBarMarvin.vi"("error in"=w1903, "Line to focus"=w1902, "reference in"=w1901) -> ("error out"=w1939:errorcluster)  [unwired: 2 out]
      n919 = property class="Tbl (strict)"(reference=w1901, error in=w1939) -> (reference out=w1920:refnum<vi>, error out=w1938:errorcluster, "Value"=w1937:string[][])
      n920 = Index Array(array=w1937, index (col)=0 ("disabled index (col)")) -> (element=w1936:string[])  [unwired: 1 in]
      n921 = call "Find_Number_LineMARVIN.vi"("Test Paragraph"=w1902, "error in"=w1938, "Row Headers[]"=w1936) -> ("error out"=w1934:errorcluster, "Line number"=w1924:i32)  [unwired: 2 in, 2 out]
      n922 = call "Table_ScrollaBarMarvin.vi"("error in"=w1934, "Line to focus"=w1902, "reference in"=w1920) -> ("error out"=w1933:errorcluster)  [unwired: 2 out]
      n923 = property class="VISAName"(reference=w1929, error in=w1933) -> (error out=w1917:errorcluster, "Value"=w1940:refnum<visa-resource-name>)  [unwired: 1 out]
      n924 = call "Wait_Sec.vi"("Delay Time (sec)"=2.0, "error out"=w1917) -> ("error in"=w1928:errorcluster)  [unwired: 2 in]
      n925 = call <vilib>:"Clear Errors.vi"("error in (no error)"=w1928) -> ("error out"=w1900:errorcluster)  [unwired: 5 in, 1 out]
      n926 = for {
        tunnel: w1940 -> [w1997]
        tunnel: w1900 -> [w1995]
        tunnel: w1921 -> [w1991] mode=indexing
        tunnel: w1920 -> [w1977]
        tunnel: w1924 -> [w1980]
        tunnel: [w1978] -> w1919
        tunnel: dbl[] [0.3, 1.7] -> [w1963] mode=indexing
        tunnel: [w1946] -> w1916 mode=indexing
        tunnel: [w1945] -> w1915 mode=indexing
        tunnel: w1905 -> [w1956]
        tunnel: w1904 -> [w1954]
        i -> [w1961]
        stop <- w1948 stop-if-true
        w1984 = 6 ("disabled index (col)")
        n927 = control-ref of="Stop Button"() -> (w1955:refnum<vi>)
        n928 = control-ref of="Motor Speed RPM"() -> (w1951:refnum<vi>)
        n929 = property on="Stop Button" class="Bool (strict)"() -> ("Value"=w1949:bool)  [unwired: 2 in, 2 out]
        n930 = Equal To 0?(x=w1961) -> (x = 0?=w1960:bool)
        n931 = Select(t="Please turn-on heat gun." ("Message"), s=w1960, f="Please turn-off heat gun." ("Message")) -> ()  [unwired: 1 out]
        n932 = Byte Array To String(unsigned byte array=w1991) -> (string=w1996:string)
        n933 = VISA Write(VISA resource name=w1997, write buffer=w1996, error in (no error)=w1995) -> (VISA resource name out=w1992:refnum<visa-resource-name>, error out=w1994:errorcluster)  [unwired: 1 out]
        n934 = flat-sequence {
          tunnel: w1957 -> [w2225]
          tunnel: [w2225] -> w1990
          tunnel: [w2224] -> w1941
          frame #0 {
            n935 = call <vilib>:"High Resolution Relative Seconds.vi"() -> ("relative seconds"=w2224:dbl)
          }
        }
        n936 = while {
          tunnel: w1941 -> [w2066]
          tunnel: w1992 -> [w2065]
          tunnel: w1990 -> [w2054]
          tunnel: [w2022] -> w1976
          tunnel: [w2013] -> w1979
          tunnel: w1961 -> [w2053]
          tunnel: [w2052] -> w1946
          tunnel: [w2032] -> w1945
          tunnel: w1963 -> [w2051]
          tunnel: w1961 -> [w2011]
          tunnel: w1956 -> [w2044]
          tunnel: w1955 -> [w2043]
          tunnel: w1954 -> [w2040]
          shift-right: [w2030] -> _
          shift-left: 0.0 ("Value") -> [w2029]
          tunnel: w1951 -> [w2026]
          shift-right: [w2019] -> _
          shift-left: 0.0 ("Value") -> [w2020]
          shift-right: [w2012] -> _
          shift-left: 0.0 ("Value") -> [w2014]
          shift-right: [w2017] -> _
          shift-left: 0.0 ("Value") -> [w2016]
          tunnel: [w2018] -> w1943
          tunnel: w1941 -> [w2015]
          stop <- w2048 stop-if-true
          w2033 = 500.0 ("y")
          # "Get Ebay fan by ADC (3)"
          n937 = control-ref of="Power transistor Heat sink Temp."() -> (w2055:refnum<vi>)
          n938 = call <vilib>:"High Resolution Relative Seconds.vi"() -> ("relative seconds"=w2056:dbl)
          n939 = Byte Array To String(unsigned byte array=u8[] [75, 0, 4, 18, 0, 0, 0, 0] ("appended array")) -> (string=w2064:string)
          n940 = VISA Write(VISA resource name=w2065, write buffer=w2064, error in (no error)=w2054) -> (VISA resource name out=w2049:refnum<visa-resource-name>, error out=w2050:errorcluster)  [unwired: 1 out]
          n941 = property on="Stop Button" class="Bool (strict)"() -> ("Value"=w2046:bool)  [unwired: 2 in, 2 out]
          n942 = Subtract(x=w2056, y=w2066) -> (x-y=w2028:dbl)
          n943 = Subtract(x=w2033, y=w2028) -> (x-y=w2038:dbl)
          n944 = Number To Fractional String(number=w2038, precision (6)=i16 2) -> (F-format string=w2037:string)  [unwired: 2 in]
          n945 = Greater Or Equal?(x=w2028, y=w2033) -> (x >= y?=w2047:bool)
          n946 = VISA Read(VISA resource name=w2049, byte count=u32 1, error in (no error)=w2050) -> (VISA resource name out=w2058:refnum<visa-resource-name>, read buffer=w2059:string, error out=w2057:errorcluster)  [unwired: 1 out]
          n947 = String To Byte Array(string=w2059) -> (unsigned byte array=w2062:u8[])
          n948 = Index Array(array=w2062, index=0) -> (element=w2060:u8)
          n949 = case shown="75" w2060 {
            tunnel: [w2167 w2173] -> w2021
            tunnel: w2058 -> [_ w2181]
            tunnel: w2057 -> [w2167 w2180]
            tunnel: [FALSE w2171] -> w2032
            tunnel: [u32 9999 w2170] -> _
            tunnel: w2051 -> [_ w2169]
            tunnel: w2011 -> [_ w2168]
            frame 0, Default {
            }
            frame 75 {
              n950 = VISA Read(VISA resource name=w2181, byte count=u32 3, error in (no error)=w2180) -> (VISA resource name out=w2176:refnum<visa-resource-name>, read buffer=w2184:string, error out=w2175:errorcluster)  [unwired: 1 out]
              n951 = String To Byte Array(string=w2184) -> (unsigned byte array=w2174:u8[])
              n952 = Index Array(array=w2174, index #1=0 ("index")) -> (element #1=w2179:u8, element #2=w2177:u8)  [unwired: 2 in, 1 out]
              n953 = Equal?(x=u8 0, y=w2179) -> (x = y?=w2178:bool)
              n954 = case shown="True" w2178 {
                tunnel: [w2187 w2195] -> w2173
                tunnel: w2177 -> [_ w2201]
                tunnel: w2176 -> [_ w2200]
                tunnel: w2175 -> [w2187 w2199]
                tunnel: w2174 -> [_ w2198]
                tunnel: [FALSE w2190] -> w2171
                tunnel: [u32 9999 w2191] -> w2170
                tunnel: w2169 -> [_ w2189]
                tunnel: w2168 -> [_ w2188]
                frame False {
                }
                frame True {
                  n955 = VISA Read(VISA resource name=w2200, byte count=w2201, error in (no error)=w2199) -> (read buffer=w2196:string, error out=w2195:errorcluster)  [unwired: 2 out]
                  n956 = String To Byte Array(string=w2196) -> (unsigned byte array=w2197:u8[])
                  n957 = Insert Into Array(array=w2198, new element=w2197) -> (w2192:u8[])  [unwired: 1 in]
                  n958 = Index Array(array=w2192, index #1=0 ("index")) -> (element #3=w2193:u8)  [unwired: 2 in, 2 out]
                  n959 = case shown="15..19" w2193 {
                    tunnel: w2192 -> [_ w2216]
                    tunnel: [u32 9999 w2207] -> w2191
                    tunnel: [FALSE w2206] -> w2190
                    tunnel: w2189 -> [_ w2205]
                    tunnel: w2188 -> [_ w2204]
                    frame 0, Default {
                    }
                    frame 15..19 {
                      n960 = Index Array(array=w2216, index #1=3 ("index")) -> (element #1=w2215:u8, element #2=w2214:u8, element #3=w2213:u8, element #4=w2212:u8)  [unwired: 3 in]
                      n961 = Join Numbers(hi=w2212, lo=w2213) -> ((hi.lo)=w2210:u16)
                      n962 = Join Numbers(hi=w2214, lo=w2215) -> ((hi.lo)=w2211:u16)
                      n963 = Join Numbers(hi=w2210, lo=w2211) -> ((hi.lo)=w2208:u32)
                      n964 = Multiply(x=0.0008056640625, y=w2208) -> (x*y=w2207:dbl)
                      n965 = case shown="0, Default" w2204 {
                        tunnel: w2207 -> [w2220 w2222]
                        tunnel: [w2219 w2221] -> w2206
                        tunnel: w2205 -> [w2218 w2223]
                        frame 0, Default {
                          n966 = Less Or Equal?(x=w2220, y=w2218) -> (x <= y?=w2219:bool)
                        }
                        frame 1 {
                          n967 = Greater Or Equal?(x=w2222, y=w2223) -> (x >= y?=w2221:bool)
                        }
                      }
                    }
                  }
                }
              }
            }
          }
          n968 = property class="DigNum (strict)"(reference=w2055, error in=w2021) -> (error out=w2023:errorcluster, "Value"=w2013:dbl)  [unwired: 1 out]
          n969 = case shown="0, Default" w2011 {
            tunnel: [w2074 FALSE] -> w2018
            tunnel: [w2073 w2129] -> w2017
            tunnel: w2016 -> [w2072 w2129]
            tunnel: w2015 -> [w2071 _]
            tunnel: w2014 -> [w2070 w2131]
            tunnel: w2013 -> [w2069 _]
            tunnel: [w2068 w2131] -> w2012
            frame 0, Default {
              n970 = disable-structure shown="Enabled" {
                disable-tunnel: w2070 -> [w2079 w2108]
                disable-tunnel: w2069 -> [w2078 w2116]
                disable-tunnel: [w2077 w2115] -> w2074
                disable-tunnel: [w2076 w2114] -> w2073
                disable-tunnel: w2072 -> [w2075 w2112]
                disable-tunnel: w2071 -> [_ _]
                disable-tunnel: w2069 -> [_ w2110]
                disable-tunnel: [_ w2109] -> w2068
                frame Disabled {
                  n971 = case shown="0, Default" {
                    selector: _ -> [_ _]
                    tunnel: w2079 -> [w2084 w2098]
                    tunnel: w2078 -> [w2083 w2097]
                    tunnel: w2075 -> [w2087 w2099]
                    tunnel: [w2086 w2100] -> w2077
                    tunnel: [w2085 w2101] -> w2076
                    frame 0, Default {
                      n972 = Subtract(x=w2083, y=w2084) -> (x-y=w2080:dbl)
                      n973 = Greater?(x=w2080, y=1.0) -> (0:w2081:bool)
                      n974 = case shown="False" w2081 {
                        tunnel: w2087 -> [w2091 _]
                        tunnel: [w2090 0.0 ("upper limit")] -> w2085
                        tunnel: [w2088 FALSE] -> w2086
                        frame False {
                          n975 = Increment(x=w2091) -> (x+1=w2090:dbl)
                          n976 = Greater Or Equal?(x=w2090, y=60.0) -> (x >= y?=w2088:bool)
                        }
                        frame True {
                        }
                      }
                    }
                    frame 1 {
                      n977 = Subtract(x=w2098, y=w2097) -> (x-y=w2096:dbl)
                      n978 = Greater?(x=w2096, y=1.0) -> (0:w2094:bool)
                      n979 = case shown="False" w2094 {
                        tunnel: w2099 -> [w2105 _]
                        tunnel: [w2104 0.0 ("upper limit")] -> w2101
                        tunnel: [w2102 FALSE] -> w2100
                        frame False {
                          n980 = Increment(x=w2105) -> (x+1=w2104:dbl)
                          n981 = Greater Or Equal?(x=w2104, y=60.0) -> (x >= y?=w2102:bool)
                        }
                        frame True {
                        }
                      }
                    }
                  }
                }
                frame Enabled {
                  n982 = Greater Or Equal?(x=w2112, y=200.0) -> (x >= y?=w2111:bool)
                  n983 = case shown="False" w2111 {
                    tunnel: w2116 -> [_ w2128]
                    tunnel: w2108 -> [_ w2127]
                    tunnel: [FALSE w2123] -> w2115
                    frame False {
                    }
                    frame True {
                      n984 = Subtract(x=w2128, y=w2127) -> (x-y=w2126:dbl)
                      n985 = Greater Or Equal?(x=w2126, y=1.0) -> (x >= y?=w2124:bool)
                      n986 = Not(x=w2124) -> (.not. x?=w2123:bool)
                    }
                  }
                  n987 = case shown="False" w2111 {
                    tunnel: [w2119 0.0] -> w2114
                    tunnel: w2112 -> [w2118 _]
                    tunnel: w2110 -> [_ w2120]
                    tunnel: [w2117 w2120] -> w2109
                    tunnel: w2108 -> [w2117 _]
                    frame False {
                      n988 = Increment(x=w2118) -> (x+1=w2119:dbl)
                    }
                    frame True {
                    }
                  }
                }
              }
            }
            frame 1 {
            }
          }
          n989 = Number To Fractional String(number=w2013, precision (6)=i16 2) -> (F-format string=w2034:string)  [unwired: 2 in]
          n990 = Concatenate Strings(w2040, "\nTimeout [sec]: " ("string"), w2037, "\nTemperature [Deg.]: " ("string"), w2034) -> (w2042:string)
          n991 = call "Write panel message (SubVI).vi"(4:"rpm"=w2026, 5:"rpm"=FALSE ("rpm"), "PrintTime"=FALSE, "Stop"=w2043, "Time to wait"=0.2, "Strin"=w2042, "String in"=w2044) -> ()  [unwired: 4 in, 1 out]
          n992 = case shown="0, Default" w2053 {
            tunnel: [w2136 w2161] -> w2052
            tunnel: w2013 -> [w2143 w2163]
            tunnel: w2032 -> [w2147 w2160]
            tunnel: [w2133 w2159] -> w2031
            tunnel: [w2143 0.0 ("Value")] -> w2030
            tunnel: w2029 -> [w2144 _]
            tunnel: w2028 -> [w2140 _]
            tunnel: [w2138 FALSE] -> w2027
            tunnel: w2023 -> [w2137 w2156]
            tunnel: [w2137 w2156] -> w2022
            tunnel: w2020 -> [w2135 w2155]
            tunnel: [w2134 w2155] -> w2019
            frame 0, Default {
              n993 = In Range and Coerce(upper limit=63.0, x=w2143, lower limit=58.0 ("y")) -> (In Range?=w2136:bool)  [unwired: 1 out]
              n994 = case shown="True" w2136 {
                tunnel: w2135 -> [_ w2154]
                tunnel: [0.0 ("Value") w2153] -> w2134
                tunnel: [FALSE w2151] -> w2132
                frame False {
                }
                frame True {
                  n995 = Increment(x=w2154) -> (x+1=w2153:dbl)
                  n996 = Greater?(x=w2153, y=15.0) -> (0:w2151:bool)
                }
              }
              n997 = Less Or Equal?(x=w2143, y=w2144) -> (x <= y?=w2142:bool)
              n998 = Greater?(x=w2140, y=200.0) -> (0:w2141:bool)
              n999 = And(x=w2142, y=w2141) -> (x .and. y?=w2138:bool)
              n1000 = Compound Arithmetic op=AND(w2136, w2147) -> (w2146:bool)
              n1001 = Or(x=w2132, y=w2146) -> (x .or. y?=w2133:bool)
            }
            frame 1 {
              n1002 = In Range and Coerce(upper limit=57.0, x=w2163, lower limit=53.0 ("y")) -> (In Range?=w2161:bool)  [unwired: 1 out]
              n1003 = Compound Arithmetic op=AND(w2161, w2160) -> (w2159:bool)
            }
          }
          n1004 = Compound Arithmetic op=OR(w2027, w2031, w2047, w2046, w2018) -> (w2048:bool)
        }
        n1005 = Number To Fractional String(number=w1979, precision (6)=i16 2) -> (F-format string=w1988:string)  [unwired: 2 in]
        n1006 = call "Write panel message (SubVI).vi"("rpm"=w1951, "PrintTime"=FALSE, "Stop"=w1955, "error in (no error)"=w1994, "Time to wait"=10.0 ("Delay Time (sec)"), "Strin"=w1954, "String in"=w1956) -> ("error out"=w1957:errorcluster)  [unwired: 4 in]
        n1007 = case shown="0, Default" w1961 {
          tunnel: w1945 -> [w2003 w2008]
          tunnel: [w2002 w2007] -> w1962
          tunnel: [w2001 FALSE] -> w1947
          tunnel: w1946 -> [w2000 _]
          tunnel: w1945 -> [w1999 _]
          frame 0, Default {
            n1008 = Not(x=w1999) -> (.not. x?=w1998:bool)
            n1009 = And(x=w2000, y=w1998) -> (x .and. y?=w2001:bool)
            n1010 = Select(t="ON", s=w2003, f="OFF") -> (s? t:f=w2002:string)
          }
          frame 1 {
            n1011 = Select(t="OFF", s=w2008, f="ON") -> (s? t:f=w2007:string)
          }
        }
        n1012 = Compound Arithmetic op=OR(w1943, w1947, w1949) -> (w1948:bool)
        n1013 = Multiply(x=w1961, y=2) -> (x*y=w1973:i32)
        n1014 = Increment(x=w1973) -> (x+1=w1974:i32)
        n1015 = Add(x=w1980, y=w1974) -> (x+y=w1975:i32)
        n1016 = call "PassOrFail (SubVI).vi"("disabled index (col)"=w1984, "index (row)"=w1975, "error in (no error)"=w1976, "Boolean"=w1946, "Table in"=w1977) -> ("error out"=w1987:errorcluster)  [unwired: 6 in]
        n1017 = property class="Tbl (strict)"(reference=w1977, error in=w1987) -> (reference out=w1968:refnum<vi>, error out=w1966:errorcluster, "Value"=w1989:string[][])
        n1018 = Replace Array Subset(array=w1989, new element=w1988, index (row)=w1975, index (col)=5 ("disabled index (col)")) -> (w1971:string[][])
        n1019 = property class="Tbl (strict)"(reference=w1968, error in=w1966, "Value"=w1971) -> (reference out=w1969:refnum<vi>, error out=w1965:errorcluster)
        n1020 = Increment(x=w1975) -> (x+1=w1985:i32)
        n1021 = call "PassOrFail (SubVI).vi"("disabled index (col)"=w1984, "index (row)"=w1985, "error in (no error)"=w1965, "Boolean"=w1945, "Table in"=w1977) -> ("error out"=w1964:errorcluster)  [unwired: 6 in]
        n1022 = property class="Tbl (strict)"(reference=w1969, error in=w1964) -> (error out=w1967:errorcluster, "Value"=w1970:string[][])  [unwired: 1 out]
        n1023 = Replace Array Subset(array=w1970, new element=w1962, index (row)=w1985, index (col)=5 ("disabled index (col)")) -> (w1986:string[][])
        n1024 = property class="Tbl (strict)"(reference=w1968, error in=w1967, "Value"=w1986) -> (error out=w1978:errorcluster)  [unwired: 1 out]
      }
      n1025 = property class="VISAName"(reference=w1929, error in=w1919) -> (error out=w1906:errorcluster, "Value"=w1932:refnum<visa-resource-name>)  [unwired: 1 out]
      n1026 = property on="Property Node" class="Bool (strict)"(error in=w1906, "DisabledEnum"=w1907) -> (error out=w1908:errorcluster)  [unwired: 1 in, 1 out]
      n1027 = property on="Property Node" class="Bool (strict)"(error in=w1908, "DisabledEnum"=w1907) -> ()  [unwired: 1 in, 2 out]
      n1028 = VISA Write(VISA resource name=w1932, write buffer=w1931, error in (no error)=w1906) -> ()  [unwired: 3 out]
      n1029 = Build Array (concatenate)(w1916, w1915) -> (w1914:bool[])
      n1030 = And Array Elements(Boolean array=w1914) -> (logical AND=→"Auxiind":bool)
    }
  }
